vi "videoAQ.vi"() -> ()   [LabVIEW 2017]
doc: "This software allows video and synchronized audio acquisition. It allows video writing to be triggered manually, by a signal to a GPIO pin on the camera, or through audio volume levels."
uses:
  <vilib>/userdefined/High Color/IMAQdx.ctl
  <vilib>/vision/driver/IMAQdx.llb/IMAQdx Attribute Type.ctl
  <vilib>/vision/Image Controls.llb/IMAQ Image.ctl
  Mux paths.ctl
  Trigger message.ctl
  <vilib>/Utility/error.llb/DialogType.ctl
  <vilib>/vision/Avi.llb/IMAQ AVI2 Refnum.ctl
  <vilib>/sound2/lvsound2.llb/Sound File Refnum.ctl
  <vilib>/sound2/lvsound2.llb/Sound Data Format.ctl
  <vilib>/vision/driver/IMAQdx.llb/IMAQdx Attribute Visibility.ctl
  <vilib>/DAQmx/write.llb/DAQmx Write (Digital Bool 1Line 1Point).vi
  <vilib>/DAQmx/read.llb/DAQmx Read (Analog Wfm 1Chan NSamp).vi
  <vilib>/DAQmx/create/channels.llb/DAQmx Create Channel (DO-Digital Output).vi
  <vilib>/DAQmx/miscellaneous.llb/DAQmx Fill In Error Info.vi
  <vilib>/DAQmx/create/channels.llb/DAQmx Create Channel (AI-Voltage-Basic).vi
  <vilib>/DAQmx/configure/timing.llb/DAQmx Timing (Sample Clock).vi
  Latest DAQmx timestamp.vi
  <vilib>/sound2/lvsound2.llb/Sound File Write Open.vi
  <vilib>/vision/driver/NI_Vision_Acquisition_Software.lvlib
  <resource>/objmgr/imaqdx.rc
  <resource>/objmgr/daqmx.rc
panel:
  out "Events and errors":string
  in  "Audio chart":enum32{"Unfiltered audio", "Filtered audio"}(tab)
  out "Unfiltered audio":waveform(dbl)(graph)
  out "Filtered audio":waveform(dbl)(graph)
  in  "Toggle debug visibility":bool
  in  "Debugging stuff":enum32{"Debug monitoring", "Camera attributes"}(tab)
  out "New triggers sent":u32
  out "Write state":T1(ring)=enum."Stopped"
  out "Video capture state":T2(ring)=enum."Stopped"
  out "Audio capture state":T2(ring)=enum."Stopped"
  out "Mux loop state":enum16{"Waiting", "Muxing", "Exiting"}(ring)
  out "Trigger out state":T3(ring)
  out "UI event loop done":bool
  out "Trigger out loop done":bool
  out "Trigger detection loop done":bool
  out "Audio capture loop done":bool
  out "Camera capture loop done":bool
  out "Video write loop done":bool
  out "Mux loop done":bool
  out "STOP":bool=TRUE
  out "dt audio trigger loop":u32
  out "Mean under low threshold for required %":bool
  out "Mean above high threshold for required %":bool
  out "Current video trigger times":T4
  out "Audio file exists":bool
  out "Video file exists":bool
  out "Updated trigger list":T5(array[cluster])
  out "Trigger updates sent":u32
  out "detecting write trigger signal":errorcluster
  out "Error after closing AVI":errorcluster
  out "Error after closing WAV":errorcluster
  out "Error after sending paths to mux loop":errorcluster
  out "Muxing error":errorcluster
  out "Dequeuing mux path error":errorcluster
  out "concatenated string":string
  out "mux path cluster":T6
  out "Attribute Information Array":T8(array[cluster])
  in  "Main controls":enum32{"Page 1"}(tab) caption="Main\ncontrols"
  in  "stop button":bool
  in  "Trigger mode":enum16{"Manual", "GPIO", "Audio"}(ring)
  in  "Capture control":enum32{"Page 1"}(tab)
  in  "Capture":bool
  in  "Enable video capture":bool=TRUE caption="Video"
  in  "Enable audio capture":bool caption="Audio"
  in  "Write control":enum32{"Page 1"}(tab)
  in  "Enable audio write":bool caption="Audio"
  in  "Enable video write":bool=TRUE caption="Video"
  in  "Trigger write to file":bool
  in  "Status":enum32{"Page 2"}(tab)
  out "Acquire framerate (fps)":dbl
  out "Video buffer":dbl(slide) scale=0.0..100.0
  out "Video buffer\n size (s)":dbl format="%_3f"
  out "Missed Frames":bool
  out "Audio buffer\nsize (s)":dbl format="%_3f"
  out "Audio buffer":dbl(slide) scale=0.0..100.0
  out "Writing video":bool
  out "Writing audio":bool
  out "Acquire sample rate (Hz)":dbl
  out "Audio buffer size (frames)":i32=5000
  in  "Settings":T9(tab)
  in  "Estimated camera latency (s)":dbl=236.0
  in  "Select camera":T10="cam0"
  in  "Frames Per Second":dbl=30.0 min=2.0 max=120.0
  in  "Audio sample rate (Hz)":i64=44100
  in  "bits per sample":i32=16
  in  "Physical channel for audio input":tag="Dev2/ai0"
  in  "Samples per\nacquisition chunk":i32=1000
  in  "Delete audio file if \ncombining is successful?":bool=TRUE
  in  "Pre-trigger time* (s)":dbl=5.0 min=0.0
  in  "Record length* (s)":dbl=10.0 min=0.0
  out "Video buffer size (frames)":i32=5000
  in  "Write directory":path
  in  "Base Filename (no extension)":string
  in  "Video codec**":string(combo)="Microsoft Video 1"
  in  "Combine audio & \nvideo into one file*":bool=TRUE
  in  "GPIO line":string(combo)="Line 0"
  in  "Low Audio Threshold %":dbl=80.0 caption="...for this \n% of..." min=0.0 max=100.0 format="%0.1f"
  in  "High Audio Threshold %":dbl=10.0 caption="...for this \n% of..." min=0.0 max=100.0 format="%0.1f"
  in  "Low Audio Threshold":dbl=0.05 caption="If audio stays \nbelow this level..." format="%0.2f"
  in  "Time cutoff (s)":dbl=20.0 caption="No matter what, stop recording \nafter this amount of time (s)"
  in  "Low monitoring period (s)":dbl=10.0 caption="...this period of time (s),\nstop the recording"
  in  "Low cutoff freq (Hz)":dbl=1000.0 format="%0.3f"
  in  "High cutoff freq (Hz)":dbl=7000.0 format="%0.3f"
  in  "High monitoring period (s)":dbl=1.0 caption="...this period of time (s), \ntrigger a recording."
  in  "High Audio Threshold":dbl=0.2 caption="If audio stays \nabove this level..." format="%0.2f"
  out "Filtered audio amplitude":T11(graph)
  out "% above high threshold":dbl format="%#.1f%"
  out "% below low threshold":dbl format="%#.1f%"
  in  "Audio trigger enable":bool=TRUE
  in  "Physical channel for trigger out":tag="Dev2/ai0"
  in  "Enable trigger out":bool
  out "Trigger out":bool
  out "Current camera session reference":T10
  out "Video input":T12(plugin-control)
  # "Video Acquisition"
  # "This is the estimated time between the camera taking an image and transmitting it to the computer. This can correct for camera latency related desyncing of audio and video."
  # "To maintain video and audio in sync, samples per acquisition * video framerate should be smaller than audio sample rate."
  # "*Applies to manual \nand GPIO trigger modes"
  # "*Requires ffmpeg"
  # "**Recommended codec:\nMicrosoft Video 1"
  # ".avi"
  # ".wav"
  # "Settings for triggering write based on GPIO input pins on the camera \n(probably will only work for Pt Grey cameras like the Flea3)"
  # "Trigger pulse should be:\n - Positive polarity (0V normally, 5V during trigger pulse)\n - At least 1/f seconds long, where f = framerate.\n - Recording will start within 1/f of the trigger receive time."
  # "Settings for triggering write based on filtered audio volume"
  # "Bandpass filter cutoffs for audio before measuring volume for triggering"
  # "Send a digital trigger out to other devices for synchronization"
  # "Trigger signal with be digital ON between recording trigger time and recording stop time, \nand digital OFF otherwise. Note that trigger signal is not ON during pre-trigger recording time."
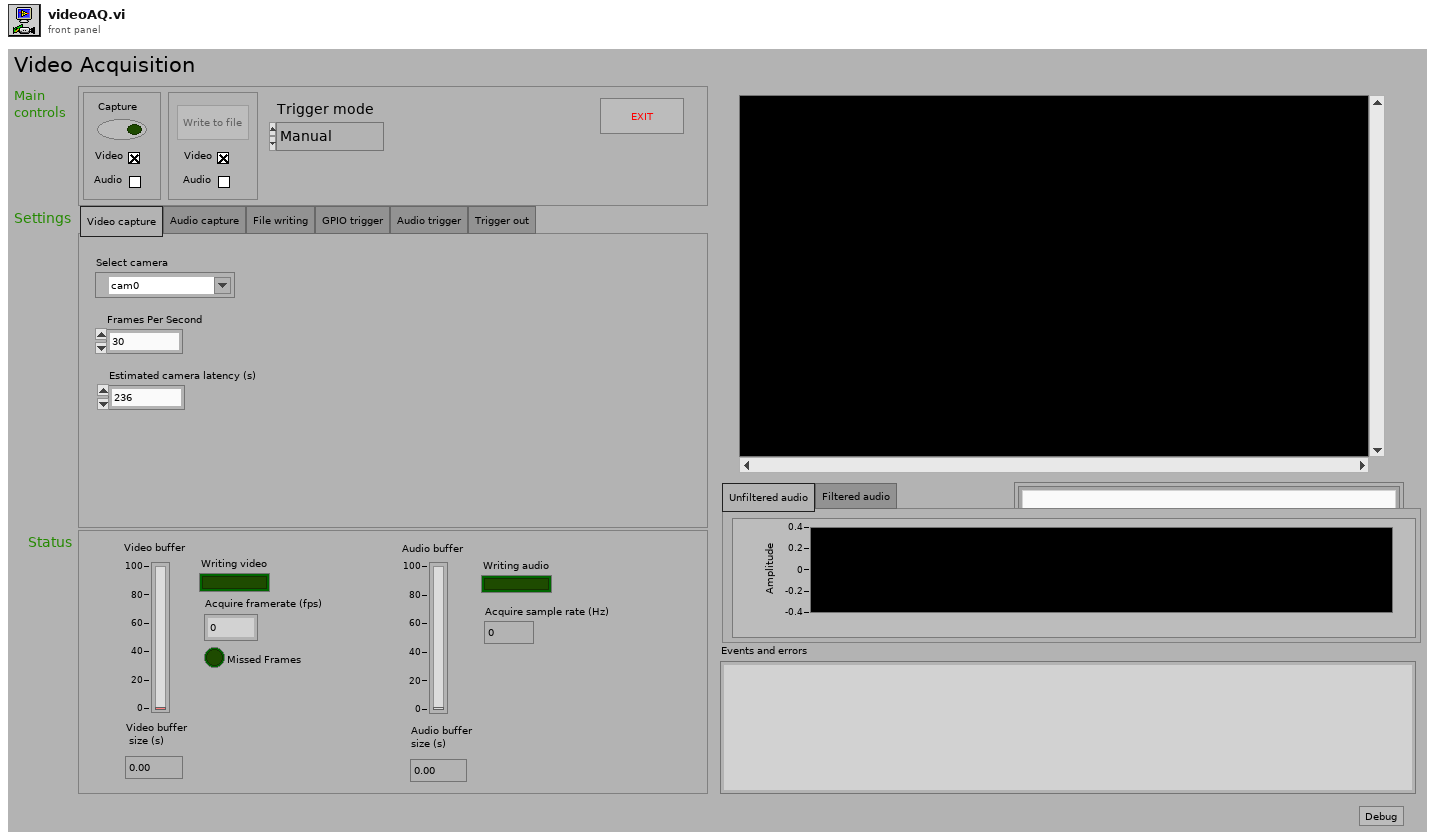
[diagram p1: front panel]
types:
  T1 = enum16{"Initializing", "Saving", "Closing file", "Stopped", "Paused", "Exiting"}
  T2 = enum16{"Initializing", "Capturing", "Stopping", "Stopped", "Exiting"}
  T3 = enum16{"Stopped", "Initializing", "Sending trigger", "Stopping", "Exiting"}
  T4 = cluster{"Start time":timestamp, "Trigger time":timestamp, "End time":timestamp}
  T5 = cluster{"Start time":timestamp, "Trigger time":timestamp, "End time":timestamp}[]
  T6 = cluster{"Available file path":path, "Available file path":path}
  T7 = typedef "NI_Vision_Acquisition_Software.lvlib/IMAQdx Attribute Type.ctl" = enum32{"U32", "I64", "DBL", "String", "Enum", "Bool", "Command"}
  T8 = cluster{"Attribute Type":T7, "Readable":bool, "Writable":bool, "Attribute Name":string}[]
  T9 = enum32{"Video capture", "Audio capture", "File writing", "GPIO trigger", "Audio trigger", "Trigger out"}
  T10 = typedef "IMAQdx.ctl" = refnum<k21>
  T11 = cluster{"Amplitude":dbl, "High Audio Threshold":dbl, "Low Audio Threshold":dbl}
  T12 = typedef "IMAQ Image.ctl" = refnum<image>
  T13 = typedef "Mux paths.ctl" = cluster{"Video path":path, "Audio path":path}
  T14 = typedef "Trigger message.ctl" = enum16{"New trigger", "Updated trigger"}
  T15 = cluster{"Trigger timestamps":cluster{"Start time":timestamp, "Trigger time":timestamp, "End time":timestamp}, "Message type":T14}
  T16 = enum16{"Always On", "Always Off", "Off While Running"}
  T17 = enum16{"At or before start", "In range", "At or after end"}
  T18 = enum16{"Stopped", "Initializing", "Sending trigger", "Stopping"}
  T19 = typedef "DialogType.ctl" = u16
  T20 = typedef "NI_Vision_Acquisition_Software.lvlib/IMAQdx Attribute Visibility.ctl" = enum32{"Simple", "Intermediate", "Advanced"}
  T21 = enum8{"Enabled", "Disabled", "Disabled and Grayed Out"}
  T22 = enum32{"Page Enabled", "Page Disabled", "Page Disabled & Grayed"}
  T23 = typedef "IMAQ AVI2 Refnum.ctl" = refnum<k20>
  T24 = typedef "Sound File Refnum.ctl" = refnum<file>
  T25 = typedef "Sound Data Format.ctl" = cluster{"sample rate (S/s)":dbl, "number of channels":i32, "bits per sample":i32}
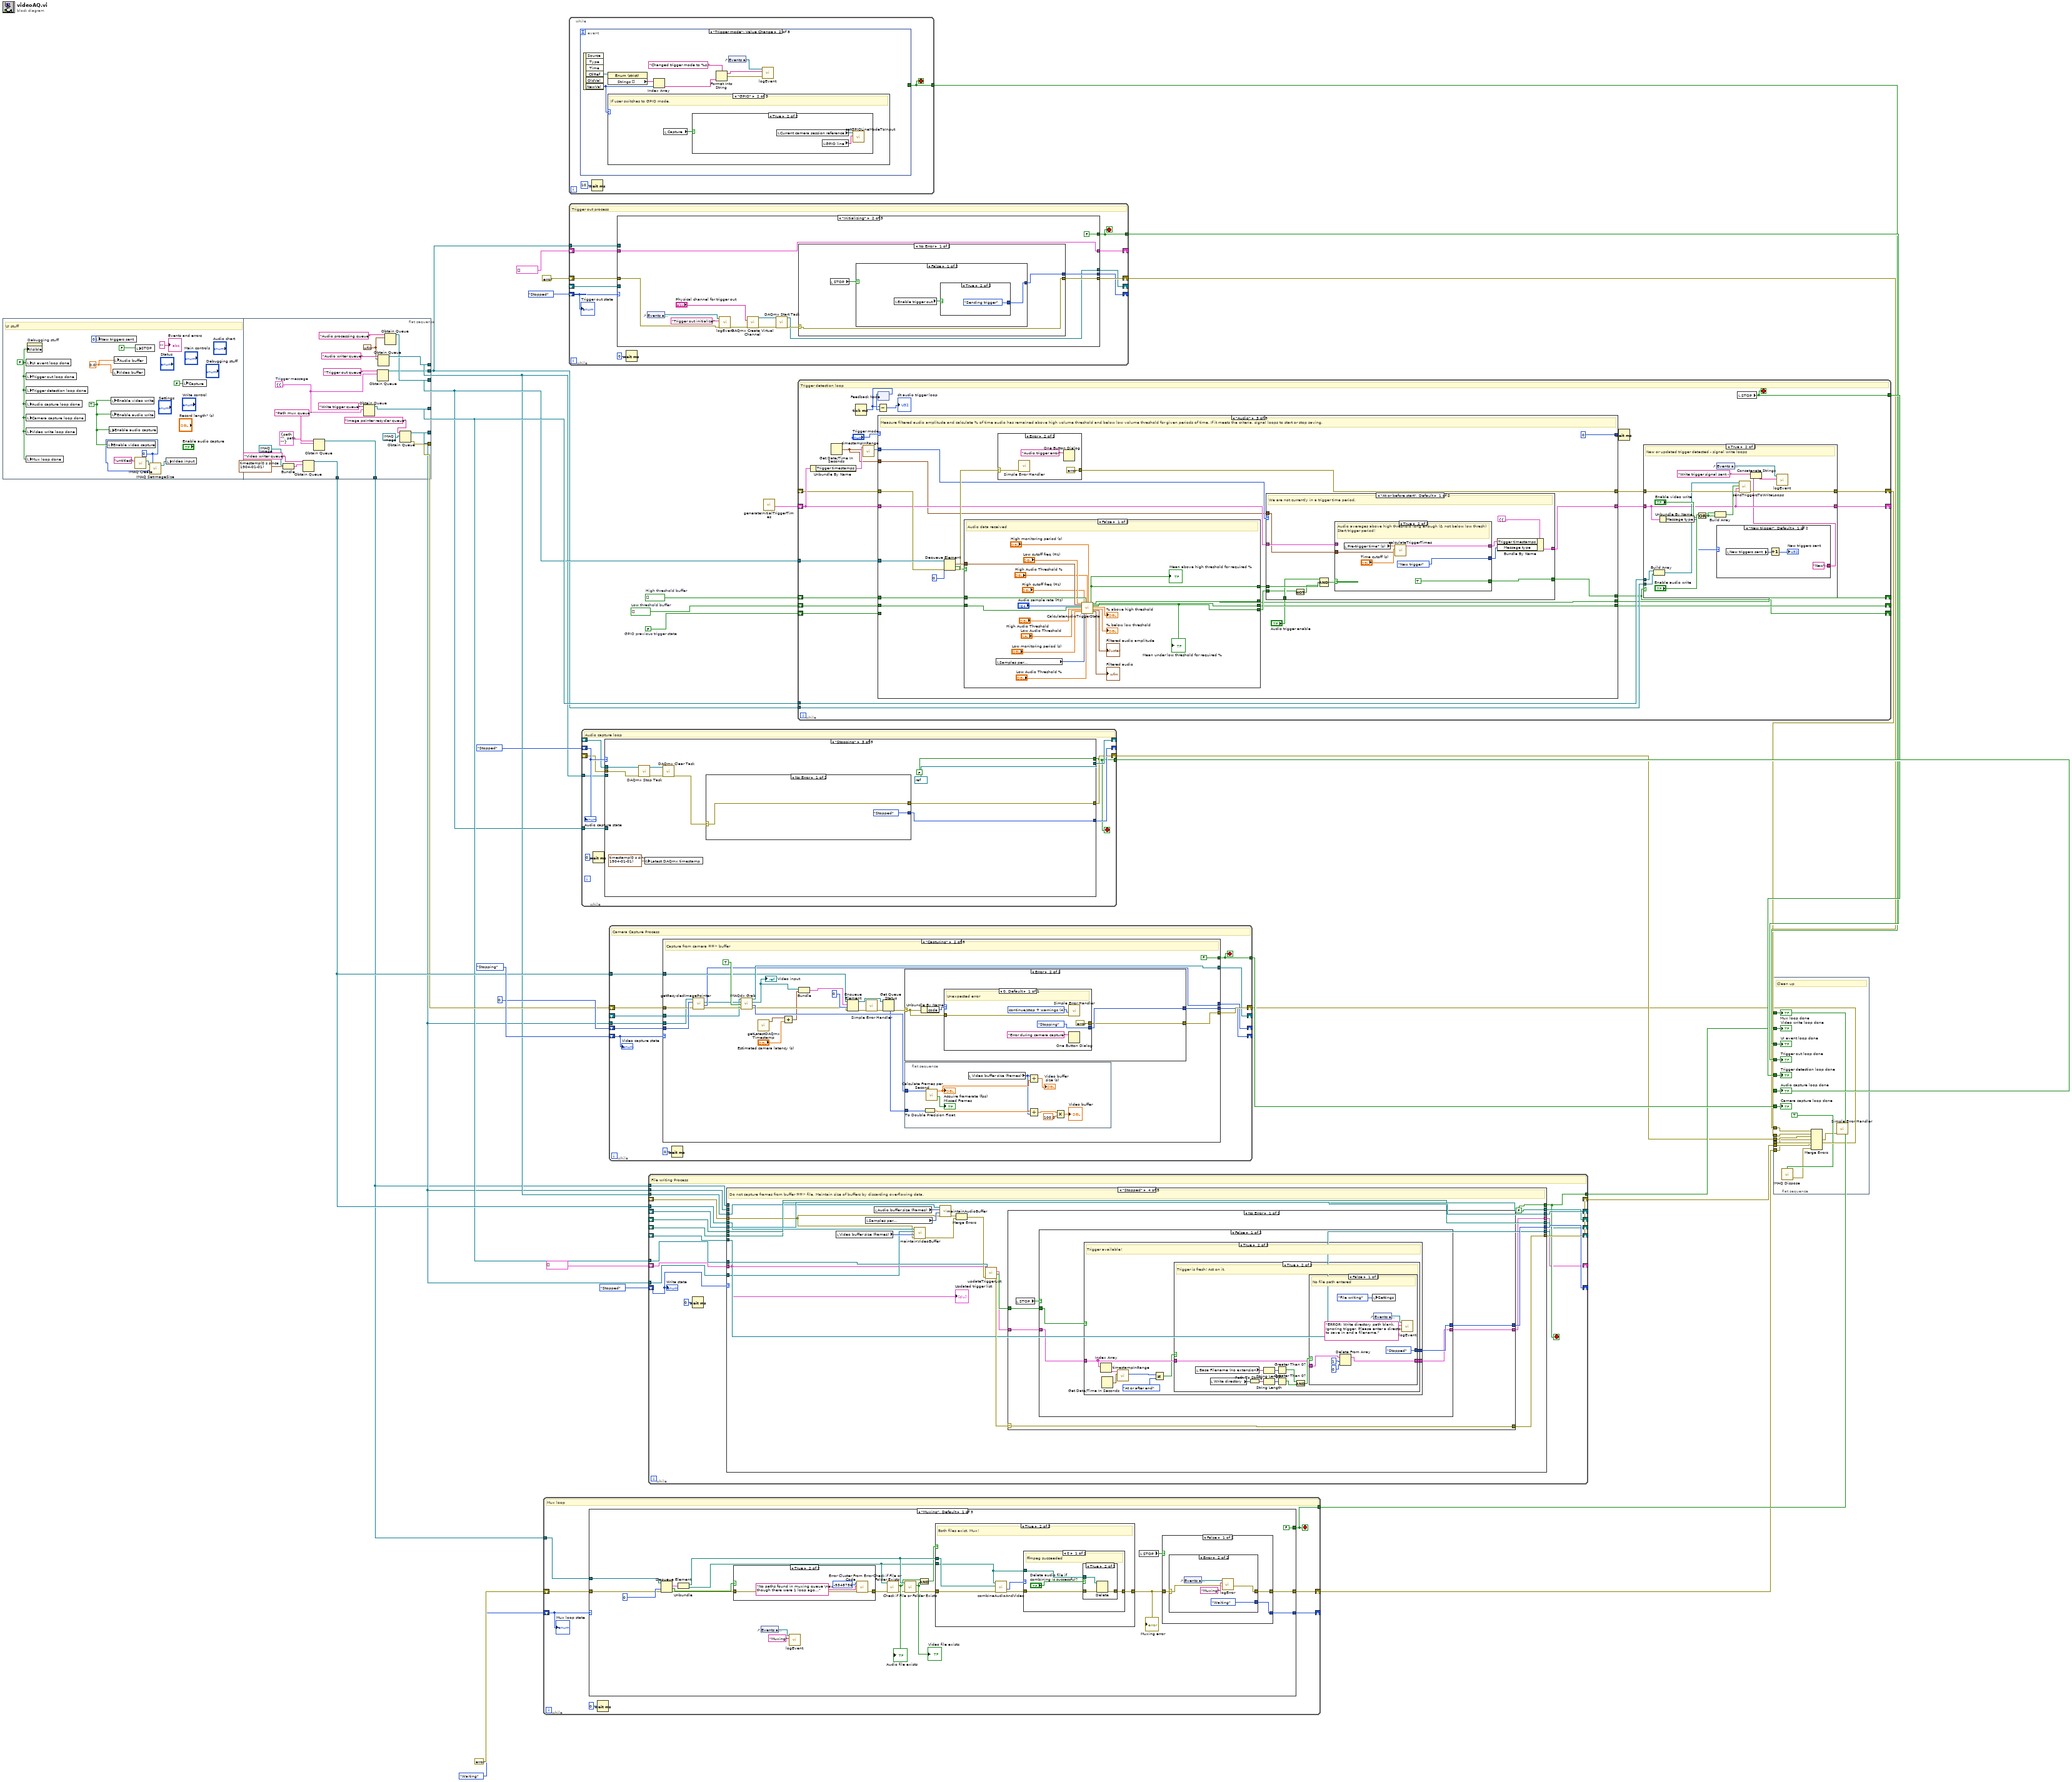
[diagram p0: block diagram]
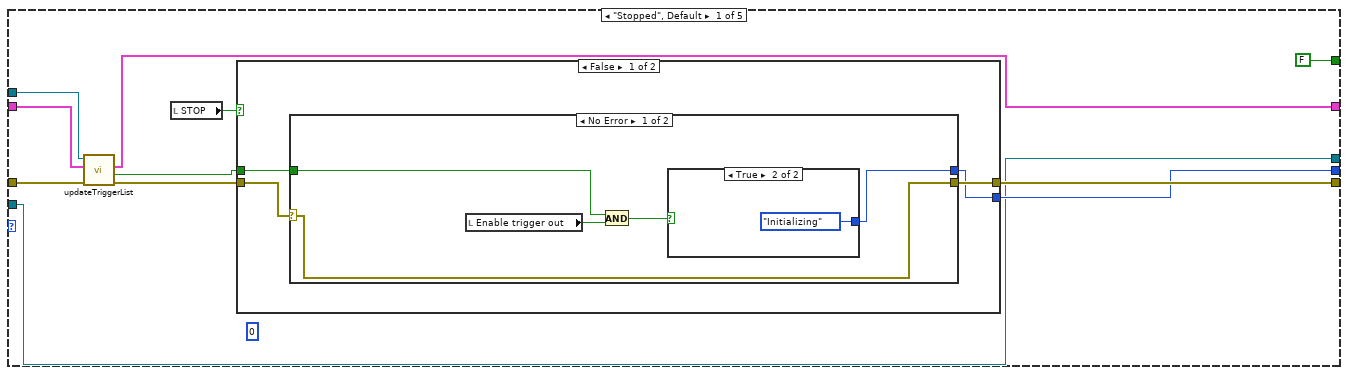
[diagram p2: hidden frame]
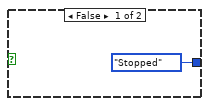
[diagram p3: hidden frame]
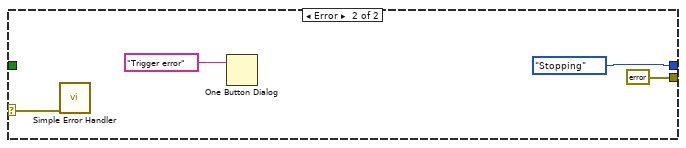
[diagram p4: hidden frame]
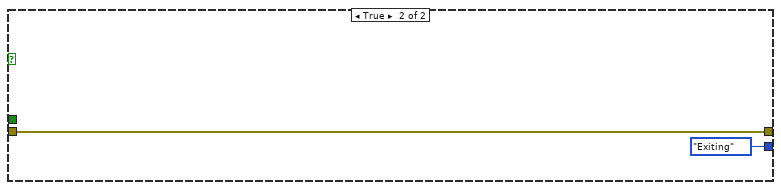
[diagram p5: hidden frame]
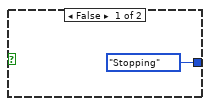
[diagram p6: hidden frame]
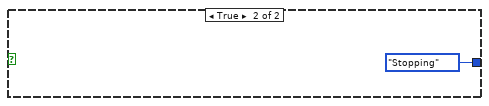
[diagram p7: hidden frame]
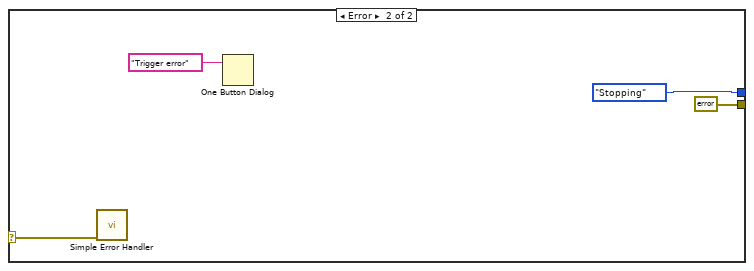
[diagram p8: hidden frame]
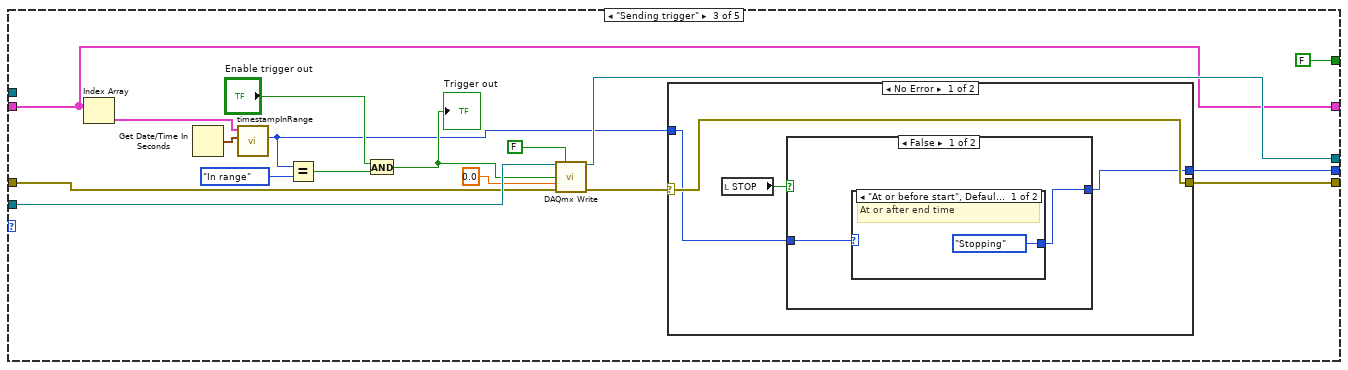
[diagram p9: hidden frame]
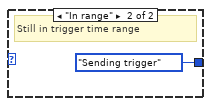
[diagram p10: hidden frame]
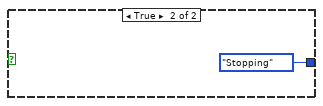
[diagram p11: hidden frame]
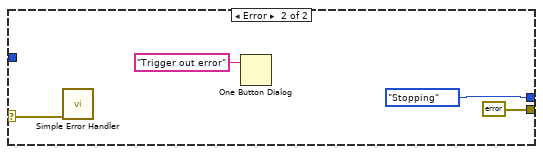
[diagram p12: hidden frame]
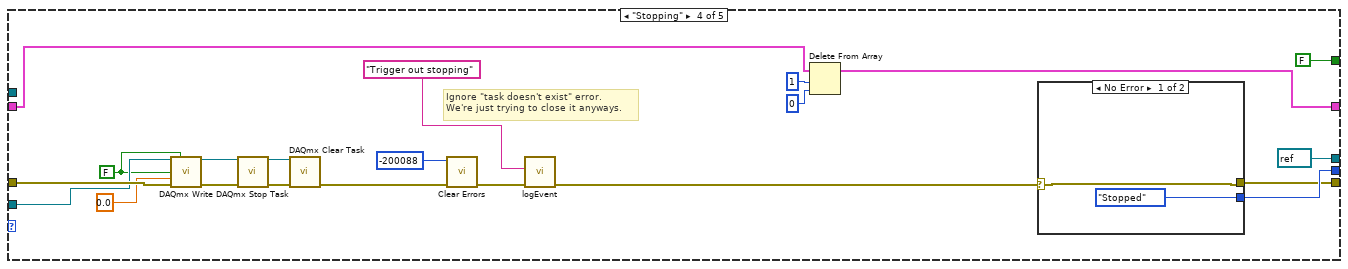
[diagram p13: hidden frame]
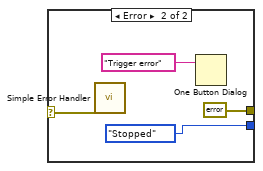
[diagram p14: hidden frame]
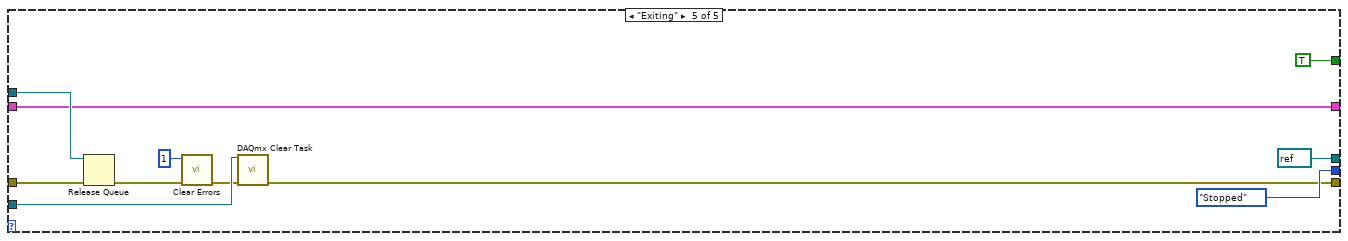
[diagram p15: hidden frame]
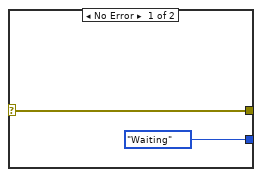
[diagram p17: hidden frame]
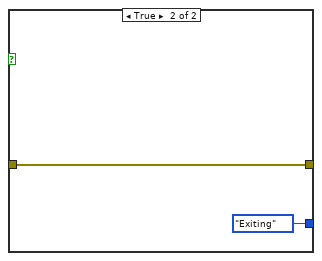
[diagram p18: hidden frame]
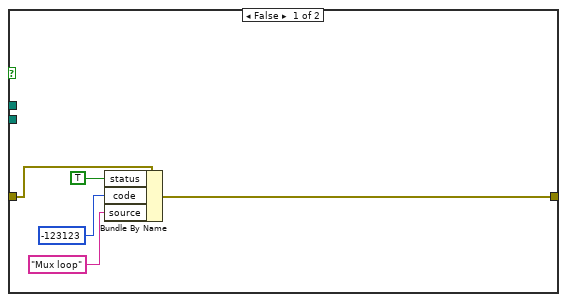
[diagram p19: hidden frame]
diagram:
  w23 = FALSE  # GPIO previous trigger state
  w24 = bool[] []  # Low threshold buffer
  w25 = bool[] []  # High threshold buffer
  n1 = flat-sequence {
    tunnel: [w66] -> w33
    tunnel: [w62] -> w31
    tunnel: [w61] -> w6
    tunnel: [w59] -> w7
    tunnel: [w57] -> w28
    tunnel: [w55] -> w29
    tunnel: [w53] -> w2
    tunnel: [w49] -> w26
    frame #0 {
      w37 = FALSE ("UI event loop done")
      w42 = 0 ("X Resolution")
      w44 = 0.0 ("Audio buffer")
      w45 = TRUE
      # "UI stuff"
      n2 = local write "UI event loop done"(w37) -> ()
      n3 = local write "Trigger out loop done"(w37) -> ()
      n4 = local write "Trigger detection loop done"(w37) -> ()
      n5 = local write "Audio capture loop done"(w37) -> ()
      n6 = local write "Camera capture loop done"(w37) -> ()
      n7 = local write "Video write loop done"(w37) -> ()
      n8 = local write "Mux loop done"(w37) -> ()
      n9 = property on="Debugging stuff" class="TabCtl (strict)"("Visible"=w37) -> ()  [unwired: 2 in, 2 out]
      n10 = local write "New triggers sent"(u32 0 ("Triggers sent")) -> ()
      n11 = local write "Enable video capture"(w45) -> ()
      n12 = local write "Enable audio capture"(w45) -> ()
      n13 = local write "Enable video write"(w45) -> ()
      n14 = local write "Enable audio write"(w45) -> ()
      n15 = local write "Video buffer"(w44) -> ()
      n16 = local write "Audio buffer"(w44) -> ()
      n17 = call "IMAQ Create"("Image Name"="untitled") -> ("New Image"=w41:T12)  [unwired: 3 in, 2 out]
      n18 = local write "STOP"(FALSE ("STOP SIGNAL")) -> ()
      n19 = call "IMAQ SetImageSize"("Y Resolution"=w42, "X Resolution"=w42, "Image"=w41) -> ("Image Out"=w40:T12)  [unwired: 2 in, 1 out]
      n20 = local write "Video input"(w40) -> ()
      n21 = local write "Capture"(FALSE ("Capture")) -> ()
      "Events and errors" <- "" ("Events and errors")
    }
    frame #1 {
      w47 = T15 {"Trigger timestamps"={"Start time"=timestamp(0 s since 1904-01-01), "Trigger time"=timestamp(0 s since 1904-01-01), "End time"=timestamp(0 s since 1904-01-01)}, "Message type"=enum."New trigger"}  # Trigger message
      w50 = waveform(dbl) {"t0"=timestamp(0 s since 1904-01-01), "dt"=1.0, "Y"=[]} ("element")
      n22 = Bundle("Image Out"=T12 refnum, timestamp(0 s since 1904-01-01)) -> (w65:cluster{"Image Out":T12, timestamp})  [unwired: 1 in]
      n23 = Obtain Queue(name (unnamed)="Video writer queue", element data type=w65) -> (queue out=w66:refnum<queue>)  [unwired: 3 in, 2 out]
      n24 = Obtain Queue(name (unnamed)="Path mux queue", element data type=T13 {"Video path"=path "", "Audio path"=path ""} ("cluster")) -> (queue out=w53:refnum<queue>)  [unwired: 3 in, 2 out]
      n25 = Obtain Queue(name (unnamed)="Write trigger queue", element data type=w47) -> (queue out=w55:refnum<queue>)  [unwired: 3 in, 2 out]
      n26 = Obtain Queue(name (unnamed)="Trigger out queue", element data type=w47) -> (queue out=w49:refnum<queue>)  [unwired: 3 in, 2 out]
      n27 = Obtain Queue(name (unnamed)="Audio writer queue", element data type=w50) -> (queue out=w59:refnum<queue>)  [unwired: 3 in, 2 out]
      n28 = Obtain Queue(name (unnamed)="Audio processing queue", element data type=w50) -> (queue out=w57:refnum<queue>)  [unwired: 3 in, 2 out]
      n29 = Obtain Queue(name (unnamed)="Image pointer recycler queue", element data type=T12 refnum ("Image Out")) -> (queue out=w61:refnum<queue>, error out=w62:errorcluster)  [unwired: 3 in, 1 out]
    }
  }
  n30 = while {
    shift-right: [w74] -> w8
    shift-left: errorcluster {"status"=FALSE, "code"=0, "source"=""} ("error IO") -> [w75]
    shift-right: [w71] -> _
    shift-left: enum16{"Waiting", "Muxing", "Exiting"}."Waiting" -> [w72]
    tunnel: [w70] -> w14
    tunnel: w2 -> [w69]
    stop <- w70 stop-if-true
    # "Mux loop"
    n31 = case shown="\"Muxing\", Default" w72 {
      tunnel: w75 -> [w78 w142 w163]
      tunnel: [w95 w146 errorcluster {"status"=FALSE, "code"=0, "source"=""} ("error IO")] -> w74
      tunnel: w69 -> [w88 w145 w165]
      tunnel: [w87 w140 enum16{"Waiting", "Muxing", "Exiting"}."Exiting"] -> w71
      tunnel: [FALSE FALSE TRUE] -> w70
      frame "Muxing", Default {
        n32 = Dequeue Element(queue=w88, timeout in ms (-1)=0, error in (no error)=w78) -> (element=w93:T13, timed out?=w80:bool, error out=w94:errorcluster)  [unwired: 1 out]
        n33 = Unbundle(w93) -> ("Video path"=w92:path, "Audio path"=w79:path)
        n34 = case shown="True" w80 {
          tunnel: w94 -> [w97 w101]
          tunnel: [w97 w100] -> w82
          frame False {
          }
          frame True {
            n35 = call <vilib>:"Error Cluster From Error Code.vi"("error in (no error)"=w101, "error message (\"\")"="No paths found in muxing queue \neven though there were 1 loop ago..." ("error message (\"\")"), "error code (0)"=-9348756) -> ("error out"=w100:errorcluster)  [unwired: 6 in]
          }
        }
        n36 = control-ref of="Events and errors"() -> (w76:refnum<vi>)
        n37 = call "logEvent.vi"("New log entry"="Muxing", "Text reference"=w76) -> ()  [unwired: 9 in, 1 out]
        n38 = call <vilib>:"Check if File or Folder Exists.vi"("error in (no error)"=w82, "path"=w79) -> ("error out"=w89:errorcluster, "file or folder exists?"=w90:bool)  [unwired: 7 in, 1 out]
        "Audio file exists" <- w90
        n39 = call <vilib>:"Check if File or Folder Exists.vi"("error in (no error)"=w89, "path"=w92) -> ("error out"=w81:errorcluster, "file or folder exists?"=w91:bool)  [unwired: 7 in, 1 out]
        "Video file exists" <- w91
        n40 = And(x=w90, y=w91) -> (x .and. y?=w85:bool)
        n41 = case shown="True" w85 {
          tunnel: w81 -> [w117 w124]
          tunnel: [w118 w120] -> w96
          tunnel: w92 -> [_ w123]
          tunnel: w79 -> [_ w119]
          frame False {
            n42 = Bundle By Name(cluster=w117, "status"=TRUE, "code"=-123123, "source"="Mux loop") -> (w118:errorcluster)
          }
          frame True {
            # "Both files exist. Mux!"
            n43 = call "combineAudioAndVideo.vi"("error in (no error)"=w124, "Video path"=w123, "Audio path"=w119) -> ("error out"=w121:errorcluster, "return code"=w122:i32)  [unwired: 7 in]
            n44 = case shown="0" w122 {
              selector: w122 -> [_ w136]
              tunnel: w121 -> [w126 w134]
              tunnel: [w125 w133] -> w120
              tunnel: w119 -> [w127 _]
              frame 0 {
                # "ffmpeg succeeded"
                n45 = case shown="True" "Delete audio file if \ncombining is successful?" {
                  tunnel: w127 -> [_ w132]
                  tunnel: w126 -> [w129 w131]
                  tunnel: [w129 w130] -> w125
                  frame False {
                  }
                  frame True {
                    n46 = Delete(path (use dialog)=w132, error in=w131) -> (error out=w130:errorcluster)  [unwired: 3 in, 2 out]
                  }
                }
              }
              frame -1, Default {
                # "ffmpeg did not succeed"
                n47 = call <vilib>:"Error Cluster From Error Code.vi"("error in (no error)"=w134, "error message (\"\")"="ffmpeg error" ("error message (\"\")"), "error code (0)"=w136) -> ("error out"=w133:errorcluster)  [unwired: 6 in]
              }
            }
          }
        }
        "Muxing error" <- w96
        n48 = local read "STOP"() -> (w84:bool)
        n49 = case shown="False" w84 {
          tunnel: w96 -> [w104 w112]
          tunnel: [w103 w112] -> w95
          tunnel: [w102 enum16{"Waiting", "Muxing", "Exiting"}."Exiting"] -> w87
          frame False {
            n50 = case shown="Error" w104 {
              selector: w104 -> [w106 w108]
              tunnel: [w106 w107] -> w103
              tunnel: [enum16{"Waiting", "Muxing", "Exiting"}."Waiting" enum16{"Waiting", "Muxing", "Exiting"}."Waiting"] -> w102
              frame No Error {
              }
              frame Error {
                n51 = control-ref of="Events and errors"() -> (w109:refnum<vi>)
                n52 = call "logError.vi"("Error to log"=w108, "Location"="Muxing", "Text reference"=w109) -> ("error out"=w107:errorcluster)  [unwired: 8 in]
              }
            }
          }
          frame True {
          }
        }
      }
      frame "Waiting" {
        # "Ignore error due to invalid queue"
        n53 = Get Queue Status(queue=w145, error in (no error)=w142) -> (error out=w138:errorcluster, # elements in queue=w144:i32)  [unwired: 1 in, 6 out]
        n54 = Greater Than 0?(x=w144) -> (x > 0?=w143:bool)
        n55 = call <vilib>:"Clear Errors.vi"("error in (no error)"=w138, "specific error code to clear (0: all)"=1) -> ("error out"=w139:errorcluster)  [unwired: 4 in, 1 out]
        "Dequeuing mux path error" <- w139
        n56 = case shown="Error" w139 {
          selector: w139 -> [w150 w157]
          tunnel: [w150 w156] -> w146
          tunnel: [w148 enum16{"Waiting", "Muxing", "Exiting"}."Waiting"] -> w140
          tunnel: w143 -> [w149 _]
          frame No Error {
            n57 = local read "STOP"() -> (w147:bool)
            n58 = case shown="False" w147 {
              tunnel: w149 -> [w152 _]
              tunnel: [w151 enum16{"Waiting", "Muxing", "Exiting"}."Exiting"] -> w148
              frame False {
                n59 = case shown="False" w152 {
                  tunnel: [enum16{"Waiting", "Muxing", "Exiting"}."Waiting" enum16{"Waiting", "Muxing", "Exiting"}."Muxing"] -> w151
                  frame False {
                    # "Haven't received audio and \nvideo paths yet. Continue waiting"
                  }
                  frame True {
                    # "Audio and video file paths received.\nBegin muxing!"
                  }
                }
              }
              frame True {
              }
            }
          }
          frame Error {
            n60 = control-ref of="Events and errors"() -> (w158:refnum<vi>)
            n61 = call "logError.vi"("Error to log"=w157, "Location"="Mux waiting", "Text reference"=w158) -> ("error out"=w156:errorcluster)  [unwired: 8 in]
          }
        }
      }
      frame "Exiting" {
        (unwired) refnum<queue> refnum ("queue out")
        n62 = Release Queue(queue=w165, force destroy? (F)=FALSE, error in (no error)=w163) -> ()  [unwired: 3 out]
      }
    }
    n63 = Wait (ms)(milliseconds to wait=u32 0) -> ()  [unwired: 1 out]
    "Mux loop state" <- w72
  }
  n64 = while {
    tunnel: [w167] -> w16
    stop <- w167 stop-if-true
    n65 = event shown="[1] \"Trigger mode\": Value Change" {
      selector: _ -> [_ _ _ _ _ _ _ _]
      dyn-events: _ -> [_ _ _ _ _ _ _ _]
      timeout: _ -> [_ _ _ _ _ _ _ _]
      tunnel: [_ _ _ w187 _ _ _ _] -> w167
      event "Enable video capture": Value Change {
        n66 = event-data() -> ("NewVal"=w169:bool)  [unwired: 1 in, 5 out]
        n67 = case shown="False" w169 {
          frame False {
            n68 = local write "Enable video write"(FALSE ("Enable video write")) -> ()
            n69 = local write "Enable audio capture"(TRUE ("Enable audio capture")) -> ()
          }
          frame True {
          }
        }
      }
      event "Trigger mode": Value Change {
        n70 = event-data() -> ("CtlRef"=w179:refnum<vi>, "NewVal"=w177:enum16{"Manual", "GPIO", "Audio"})  [unwired: 1 in, 4 out]
        n71 = property class="Enum (strict)"(reference=w179) -> ("Strings []"=w178:string[])  [unwired: 1 in, 2 out]
        n72 = case shown="\"GPIO\"" w177 {
          frame "Manual", Default {
          }
          frame "GPIO" {
            # "If user switches to GPIO mode,"
            n73 = local read "Capture"() -> (w180:bool)
            n74 = case shown="True" w180 {
              frame False {
              }
              frame True {
                n75 = local read "Current camera session reference"() -> (w182:T10)
                n76 = local read "GPIO line"() -> (w181:string)
                n77 = call "setGPIOLineModeToInput.vi"("GPIO line"=w181, "IMAQdx Session in"=w182) -> ()  [unwired: 8 in, 2 out]
              }
            }
          }
          frame "Audio" {
            n78 = local write "Enable audio capture"(TRUE ("Enable audio capture")) -> ()
          }
        }
        n79 = Index Array(array=w178, index=w177) -> (element=w173:string)
        n80 = Format Into String(format string="Changed trigger mode to %s.", w173) -> (resulting string=w175:string, error out=w174:errorcluster)  [unwired: 2 in]
        n81 = control-ref of="Events and errors"() -> (w172:refnum<vi>)
        n82 = call "logEvent.vi"("error in (no error)"=w174, "New log entry"=w175, "Text reference"=w172) -> ()  [unwired: 8 in, 1 out]
      }
      event "High Audio Threshold": Value Change {
        n83 = event-data() -> ("NewVal"=w186:dbl)  [unwired: 1 in, 5 out]
        n84 = Multiply(x=1.5, y=w186) -> (x*y=w184:dbl)
        n85 = property on="Filtered audio amplitude" class="WFChart (strict)"("YScale.Maximum"=w184) -> ()  [unwired: 2 in, 2 out]
      }
      event "stop button": Value Change {
        n86 = event-data() -> ()  [unwired: 1 in, 6 out]
        n87 = case shown="True" "stop button" {
          tunnel: [FALSE ("STOP SIGNAL") w190] -> w187
          frame False {
          }
          frame True {
            w190 = TRUE ("STOP SIGNAL")
            # "Set stop signal to true"
            "STOP" <- w190
          }
        }
      }
      event "Toggle debug visibility": Value Change {
        n88 = event-data() -> ()  [unwired: 1 in, 6 out]
        n89 = property on="Debugging stuff" class="TabCtl (strict)"() -> ("Visible"=w197:bool)  [unwired: 2 in, 2 out]
        n90 = Not(x=w197) -> (.not. x?=w192:bool)
        n91 = case shown="False" w192 {
          tunnel: [T16."Always Off" ("Horizontal Scrollbar Visibility") T16."Always On" ("Horizontal Scrollbar Visibility")] -> w191
          frame False {
          }
          frame True {
          }
        }
        n92 = property on="Debugging stuff" class="TabCtl (strict)"("Visible"=w192) -> ()  [unwired: 2 in, 2 out]
        n93 = property class="VI"() -> ("Panel"=w194:refnum<vi>)  [unwired: 2 in, 2 out]
        n94 = property class="Pnl"(reference=w194) -> ("Panes[]"=w195:refnum<vi>[])  [unwired: 1 in, 2 out]
        n95 = Index Array(array=w195) -> (element=w196:refnum<vi>)  [unwired: 1 in]
        n96 = property class="Pane"(reference=w196, "HorizScrollbarVisibility"=w191) -> ()  [unwired: 1 in, 2 out]
        n97 = property class="Pane"(reference=w196, "VertScrollbarVisibility"=w191) -> (reference out=w193:refnum<vi>)  [unwired: 1 in, 1 out]
        n98 = Close Reference(reference=w193) -> ()  [unwired: 1 in, 1 out]
      }
      event "Enable audio capture": Value Change {
        n99 = event-data() -> ("NewVal"=w200:bool)  [unwired: 1 in, 5 out]
        n100 = case shown="False" w200 {
          frame False {
            n101 = local write "Enable audio write"(FALSE ("Enable video write")) -> ()
            n102 = local write "Enable video capture"(TRUE ("Enable video capture")) -> ()
          }
          frame True {
          }
        }
      }
      event "Enable video write": Value Change {
        n103 = event-data() -> ("NewVal"=w203:bool)  [unwired: 1 in, 5 out]
        n104 = case shown="True" w203 {
          frame False {
            n105 = local write "Enable audio write"(TRUE ("Enable audio write")) -> ()
          }
          frame True {
            n106 = local write "Enable video capture"(TRUE ("Enable video capture")) -> ()
          }
        }
      }
      event "Enable audio write": Value Change {
        n107 = event-data() -> ("NewVal"=w206:bool)  [unwired: 1 in, 5 out]
        n108 = case shown="True" w206 {
          frame False {
            # "If audio write is set to false, set video write to true"
            n109 = local write "Enable video write"(TRUE ("Enable video write")) -> ()
          }
          frame True {
            # "If audio write is set to true, set audio capture to true too"
            n110 = local write "Enable audio capture"(TRUE ("Enable audio capture")) -> ()
          }
        }
      }
    }
    n111 = Wait (ms)(milliseconds to wait=u32 10) -> ()  [unwired: 1 out]
  }
  n112 = while {
    shift-right: [w218] -> w13
    shift-left: errorcluster {"status"=FALSE, "code"=0, "source"=""} ("error IO") -> [w219]
    shift-right: [w217] -> _
    shift-left: _ -> [w216]
    tunnel: w26 -> [w215]
    shift-right: [w209] -> _
    shift-left: T5 [] -> [w210]
    shift-right: [w212] -> _
    shift-left: T3."Stopped" -> [w213]
    tunnel: [w211] -> w17
    stop <- w211 stop-if-true
    # "Trigger out process"
    n113 = case shown="\"Initializing\"" w213 {
      tunnel: w219 -> [w223 w251 w287 w315 w337]
      tunnel: [w230 w259 w285 w322 w334] -> w218
      tunnel: [w229 w260 w284 w323 T3."Stopped"] -> w212
      tunnel: [w228 w254 w288 refnum<k21> refnum ("task out") refnum<k21> refnum ("task out")] -> w217
      tunnel: w216 -> [w228 _ w289 w313 w336]
      tunnel: w215 -> [w224 _ _ _ w338]
      tunnel: [FALSE FALSE FALSE FALSE TRUE] -> w211
      tunnel: w210 -> [w225 w252 w280 w307 w330]
      tunnel: [w220 w252 w280 w306 w330] -> w209
      frame "Stopped", Default {
        (unwired) 0 ("timeout in ms (-1)")
        n114 = call "updateTriggerList.vi"("error in (no error)"=w223, "Trigger list"=w225, "Trigger queue in"=w224) -> ("error out"=w221:errorcluster, "Trigger available?"=w222:bool, "Updated trigger list"=w220:T5)  [unwired: 5 in, 1 out]
        n115 = local read "STOP"() -> (w226:bool)
        n116 = case shown="False" w226 {
          tunnel: [w234 w246] -> w230
          tunnel: [w233 T3."Exiting"] -> w229
          tunnel: w222 -> [w232 _]
          tunnel: w221 -> [w231 w246]
          frame False {
            n117 = case shown="No Error" w231 {
              selector: w231 -> [w239 w245]
              tunnel: [w239 errorcluster {"status"=FALSE, "code"=0, "source"=""} ("error IO")] -> w234
              tunnel: [w238 T3."Stopping"] -> w233
              tunnel: w232 -> [w235 _]
              frame No Error {
                n118 = local read "Enable trigger out"() -> (w237:bool)
                n119 = And(x=w235, y=w237) -> (x .and. y?=w236:bool)
                n120 = case shown="True" w236 {
                  tunnel: [T3."Stopped" T3."Initializing"] -> w238
                  frame False {
                  }
                  frame True {
                  }
                }
              }
              frame Error {
                n121 = call <vilib>:"Simple Error Handler.vi"("error in (no error)"=w245) -> ()  [unwired: 4 in, 5 out]
                n122 = One Button Dialog(message="Trigger error") -> ()  [unwired: 1 in, 1 out]
              }
            }
          }
          frame True {
          }
        }
      }
      frame "Initializing" {
        n123 = control-ref of="Events and errors"() -> (w248:refnum<vi>)
        n124 = call "logEvent.vi"("error in (no error)"=w251, "New log entry"="Trigger out initialize", "Text reference"=w248) -> ("error out"=w250:errorcluster)  [unwired: 8 in]
        n125 = call-poly <vilib>:"DAQmx Create Virtual Channel.vi"("lines"="Physical channel for trigger out", "error in"=w250) -> ("task out"=w256:refnum<k21>, "error out"=w257:errorcluster)  [unwired: 12 in]
        n126 = call <vilib>:"DAQmx Start Task.vi"("task/channels in"=w256, "error in"=w257) -> ("task out"=w254:refnum<k21>, "error out"=w255:errorcluster)  [unwired: 12 in]
        n127 = case shown="No Error" w255 {
          selector: w255 -> [w263 w272]
          tunnel: [w263 errorcluster {"status"=FALSE, "code"=0, "source"=""} ("error IO")] -> w259
          tunnel: [w262 T3."Stopping"] -> w260
          frame No Error {
            n128 = local read "STOP"() -> (w261:bool)
            n129 = case shown="False" w261 {
              tunnel: [w265 T3."Stopping"] -> w262
              frame False {
                n130 = local read "Enable trigger out"() -> (w264:bool)
                n131 = case shown="True" w264 {
                  tunnel: [T3."Stopping" T3."Sending trigger"] -> w265
                  frame False {
                  }
                  frame True {
                  }
                }
              }
              frame True {
              }
            }
          }
          frame Error {
            n132 = call <vilib>:"Simple Error Handler.vi"("error in (no error)"=w272) -> ()  [unwired: 4 in, 5 out]
            n133 = One Button Dialog(message="Trigger error") -> ()  [unwired: 1 in, 1 out]
          }
        }
      }
      frame "Sending trigger" {
        n134 = Index Array(array=w280) -> (element=w279:T4)  [unwired: 1 in]
        n135 = Get Date/Time In Seconds() -> (seconds since 1Jan1904=w277:timestamp)
        n136 = call "timestampInRange.vi"("Time Stamp"=w277, "Start and end times"=w279) -> ("timeState"=w273:T17)  [unwired: 9 in]
        n137 = Equal?(x=w273, y=T17."In range") -> (x = y?=w274:bool)
        n138 = And(x="Enable trigger out", y=w274) -> (x .and. y?=w275:bool)
        "Trigger out" <- w275
        n139 = call-poly <vilib>:"DAQmx Write.vi"("task/channels in"=w289, "auto start"=FALSE, "data"=w275, "timeout"=0.0, "error in"=w287) -> ("task out"=w288:refnum<k21>, "error out"=w286:errorcluster)  [unwired: 8 in, 1 out]
        n140 = case shown="No Error" w286 {
          selector: w286 -> [w293 w302]
          tunnel: [w293 errorcluster {"status"=FALSE, "code"=0, "source"=""} ("error IO")] -> w285
          tunnel: [w292 T18."Stopping"] -> w284
          tunnel: w273 -> [w290 _]
          frame No Error {
            n141 = local read "STOP"() -> (w291:bool)
            n142 = case shown="False" w291 {
              tunnel: [w295 T3."Stopping"] -> w292
              tunnel: w290 -> [w294 _]
              frame False {
                n143 = case shown="\"At or before start\", Default" w294 {
                  tunnel: [T3."Stopping" T3."Sending trigger"] -> w295
                  frame "At or before start", Default {
                    # "At or after end time"
                  }
                  frame "In range" {
                    # "Still in trigger time range"
                  }
                }
              }
              frame True {
              }
            }
          }
          frame Error {
            n144 = call <vilib>:"Simple Error Handler.vi"("error in (no error)"=w302) -> ()  [unwired: 4 in, 5 out]
            n145 = One Button Dialog(message="Trigger out error") -> ()  [unwired: 1 in, 1 out]
          }
        }
      }
      frame "Stopping" {
        w311 = FALSE ("auto start")
        # "Ignore \"task doesn't exist\" error.\nWe're just trying to close it anyways."
        n146 = call-poly <vilib>:"DAQmx Write.vi"("task/channels in"=w313, "auto start"=w311, "data"=w311, "timeout"=0.0, "error in"=w315) -> ("task out"=w312:refnum<k21>, "error out"=w314:errorcluster)  [unwired: 8 in, 1 out]
        n147 = call <vilib>:"DAQmx Stop Task.vi"("task/channels in"=w312, "error in"=w314) -> ("task out"=w321:refnum<k21>, "error out"=w320:errorcluster)  [unwired: 12 in]
        n148 = call <vilib>:"DAQmx Clear Task.vi"("task in"=w321, "error in"=w320) -> ("error out"=w319:errorcluster)  [unwired: 13 in]
        n149 = call <vilib>:"Clear Errors.vi"("error in (no error)"=w319, "specific error code to clear (0: all)"=-200088) -> ("error out"=w304:errorcluster)  [unwired: 4 in, 1 out]
        n150 = call "logEvent.vi"("error in (no error)"=w304, "New log entry"="Trigger out stopping") -> ("error out"=w303:errorcluster)  [unwired: 9 in]
        n151 = Delete From Array(array=w307, length=1, index=0) -> (array with subset deleted=w306:T5)  [unwired: 1 out]
        n152 = case shown="No Error" w303 {
          selector: w303 -> [w325 w327]
          tunnel: [w325 errorcluster {"status"=FALSE, "code"=0, "source"=""} ("error IO")] -> w322
          tunnel: [T3."Stopped" T3."Stopped"] -> w323
          frame No Error {
          }
          frame Error {
            n153 = call <vilib>:"Simple Error Handler.vi"("error in (no error)"=w327) -> ()  [unwired: 4 in, 5 out]
            n154 = One Button Dialog(message="Trigger error") -> ()  [unwired: 1 in, 1 out]
          }
        }
      }
      frame "Exiting" {
        n155 = Release Queue(queue=w338, error in (no error)=w337) -> (error out=w335:errorcluster)  [unwired: 1 in, 2 out]
        n156 = call <vilib>:"Clear Errors.vi"("error in (no error)"=w335, "specific error code to clear (0: all)"=1) -> ("error out"=w332:errorcluster)  [unwired: 4 in, 1 out]
        n157 = call <vilib>:"DAQmx Clear Task.vi"("task in"=w336, "error in"=w332) -> ("error out"=w334:errorcluster)  [unwired: 13 in]
      }
    }
    n158 = Wait (ms)(milliseconds to wait=u32 0) -> ()  [unwired: 1 out]
    "Trigger out state" <- w213
  }
  n159 = while {
    tunnel: w7 -> [w346]
    shift-right: [w344] -> _
    shift-left: T2."Stopped" -> [w350]
    shift-right: [w345] -> w11
    shift-left: _ -> [w349]
    shift-right: [w348] -> _
    shift-left: _ -> [w347]
    tunnel: w28 -> [w343]
    tunnel: [w341] -> w19
    stop <- w341 stop-if-true
    # "Audio capture loop"
    n160 = Wait (ms)(milliseconds to wait=u32 0) -> ()  [unwired: 1 out]
    n161 = case shown="\"Stopping\"" w350 {
      tunnel: [FALSE FALSE FALSE FALSE TRUE] -> w341
      tunnel: w349 -> [w361 w404 w442 w458 w469]
      tunnel: [w360 w405 refnum<k21> refnum ("task out") refnum<k21> refnum ("task out") refnum<k21> refnum ("task out")] -> w348
      tunnel: w347 -> [_ w406 w443 _ _]
      tunnel: w346 -> [_ w403 _ _ w471]
      tunnel: [w351 w396 w440 w458 w468] -> w345
      tunnel: [w352 w397 w439 w457 T2."Exiting"] -> w344
      tunnel: w343 -> [_ w394 _ _ _]
      frame "Initializing", Default {
        w372 = 10083 items=["default"=-1, "RSE"=10083, "NRSE"=10078, "Differential"=10106, "Pseudodifferential"=12529] ("Terminal Configuration")
        w376 = 10123 items=["Finite Samples"=10178, "Continuous Samples"=10123, "Hardware Timed Single Point"=12522]  # Sample Mode
        n162 = local read "Audio sample rate (Hz)"() -> (w368:i64)
        n163 = call-poly <vilib>:"DAQmx Create Virtual Channel.vi"("maximum value"=10.0 ("Max Voltage"), "minimum value"=-10.0 ("Min Voltage"), "input terminal configuration"=w372, "physical channels"="Physical channel for audio input", "error in"=w361) -> ("task out"=w374:refnum<k21>, "error out"=w375:errorcluster)  [unwired: 9 in]
        n164 = call-poly <vilib>:"DAQmx Timing.vi"("task/channels in"=w374, "sample mode"=w376, "samples per channel"="Samples per\nacquisition chunk", "rate"=w368, "source"=tag "OnboardClock" ("Sample Clock Source"), "error in"=w375) -> ("task out"=w366:refnum<k21>, "error out"=w365:errorcluster)  [unwired: 8 in]
        n165 = local read "Audio sample rate (Hz)"() -> (w356:i64)
        n166 = local read "Pre-trigger time* (s)"() -> (w357:dbl)
        n167 = property class="DAQmx Timing"(reference=w366, error in=w365) -> (reference out=w363:refnum<k21>, error out=w362:errorcluster, "SampClk.Rate"=→"Acquire sample rate (Hz)":dbl)
        n168 = Increment(x=w357) -> (x+1=w358:dbl)
        n169 = call <vilib>:"DAQmx Start Task.vi"("task/channels in"=w363, "error in"=w362) -> ("task out"=w360:refnum<k21>, "error out"=w359:errorcluster)  [unwired: 12 in]
        n170 = Multiply(x=w356, y=w358) -> (x*y=w355:dbl)
        n171 = Round Toward +Infinity(x=w355) -> (ceil(x): smallest int >= x=w354:dbl)
        n172 = To Long Integer(number=w354) -> (32bit integer=→"Audio buffer size (frames)":i32)
        n173 = case shown="No Error" w359 {
          selector: w359 -> [w379 w387]
          tunnel: [w380 T2."Stopping"] -> w352
          tunnel: [w379 errorcluster {"status"=FALSE, "code"=0, "source"=""} ("error IO")] -> w351
          frame No Error {
            n174 = local read "STOP"() -> (w378:bool)
            n175 = case shown="True" w378 {
              tunnel: [T2."Capturing" T2."Stopping"] -> w380
              frame False {
              }
              frame True {
              }
            }
          }
          frame Error {
            n176 = call <vilib>:"Simple Error Handler.vi"("error in (no error)"=w387) -> ()  [unwired: 4 in, 5 out]
            n177 = local write "Settings"(T9."Video capture" ("Settings")) -> ()
            n178 = One Button Dialog(message="Error in audio\ncapture initialization.\nDisabling audio capture.") -> ()  [unwired: 1 in, 1 out]
            n179 = local write "Enable audio capture"(FALSE ("Enable audio capture")) -> ()
          }
        }
      }
      frame "Capturing" {
        n180 = local read "Samples per\nacquisition chunk"() -> (w398:i32)
        n181 = call-poly <vilib>:"DAQmx Read.vi"("task/channels in"=w406, "number of samples per channel"=w398, "error in"=w404) -> ("task out"=w405:refnum<k21>, "data"=w390:waveform(dbl), "error out"=w402:errorcluster)  [unwired: 10 in]
        "Unfiltered audio" <- w390
        n182 = Enqueue Element(queue=w403, element=w390, timeout in ms (-1)=0, error in (no error)=w402) -> (queue out=w400:refnum<queue>, error out=w393:errorcluster)  [unwired: 1 out]
        n183 = Unbundle By Name(w390) -> ("t0"=w389:timestamp)
        n184 = Get Queue Status(queue=w400, error in (no error)=w393) -> (error out=w392:errorcluster, # elements in queue=w399:i32)  [unwired: 1 in, 6 out]
        n185 = global write "Latest DAQmx timestamp.vi" "Latest DAQmx timestamp"(w389) -> ()
        n186 = local read "Trigger mode"() -> (w395:enum16{"Manual", "GPIO", "Audio"})
        n187 = flat-sequence {
          tunnel: w399 -> [w419]
          frame #0 {
            n188 = local read "Samples per\nacquisition chunk"() -> (w416:i32)
            n189 = local read "Audio sample rate (Hz)"() -> (w418:i64)
            n190 = local read "Audio buffer size (frames)"() -> (w415:i32)
            n191 = Multiply(x=w419, y=w416) -> (x*y=w417:i32)
            n192 = To Double Precision Float(number=w417) -> (double precision float=w420:dbl)
            n193 = Divide(x=w415, y=w418) -> (x/y=→"Audio buffer\nsize (s)":dbl)
            n194 = Divide(x=w420, y=w415) -> (x/y=w423:dbl)
            n195 = Multiply(x=w423, y=100.0) -> (x*y=→"Audio buffer":dbl)
          }
        }
        n196 = case shown="\"Audio\"" w395 {
          tunnel: w394 -> [_ _ w413]
          tunnel: w390 -> [_ _ w412]
          tunnel: w392 -> [w408 w409 w411]
          tunnel: [w408 w409 w410] -> w391
          frame "Manual", Default {
          }
          frame "GPIO" {
          }
          frame "Audio" {
            # "If trigger mode is audio, send efference copy of audio to processing loop"
            n197 = Enqueue Element(queue=w413, element=w412, error in (no error)=w411) -> (error out=w410:errorcluster)  [unwired: 1 in, 2 out]
          }
        }
        n198 = case shown="No Error" w391 {
          selector: w391 -> [w425 w436]
          tunnel: [w426 T2."Stopping"] -> w397
          tunnel: [w425 errorcluster {"status"=FALSE, "code"=0, "source"=""} ("error IO")] -> w396
          frame No Error {
            n199 = local read "STOP"() -> (w424:bool)
            n200 = case shown="True" w424 {
              tunnel: [w430 T2."Stopping"] -> w426
              frame False {
                n201 = local read "Enable audio capture"() -> (w429:bool)
                n202 = local read "Capture"() -> (w428:bool)
                n203 = And(x=w428, y=w429) -> (x .and. y?=w427:bool)
                n204 = case shown="True" w427 {
                  tunnel: [T2."Stopping" T2."Capturing"] -> w430
                  frame False {
                  }
                  frame True {
                  }
                }
              }
              frame True {
              }
            }
          }
          frame Error {
            n205 = call <vilib>:"Simple Error Handler.vi"("error in (no error)"=w436) -> ()  [unwired: 4 in, 5 out]
            n206 = One Button Dialog(message="Error in audio capture") -> ()  [unwired: 1 in, 1 out]
          }
        }
      }
      frame "Stopping" {
        n207 = call <vilib>:"DAQmx Stop Task.vi"("task/channels in"=w443, "error in"=w442) -> ("task out"=w444:refnum<k21>, "error out"=w445:errorcluster)  [unwired: 12 in]
        n208 = global write "Latest DAQmx timestamp.vi" "Latest DAQmx timestamp"(timestamp(0 s since 1904-01-01) ("Latest DAQmx timestamp")) -> ()
        n209 = call <vilib>:"DAQmx Clear Task.vi"("task in"=w444, "error in"=w445) -> ("error out"=w441:errorcluster)  [unwired: 13 in]
        n210 = case shown="No Error" w441 {
          selector: w441 -> [w449 w454]
          tunnel: [w449 errorcluster {"status"=FALSE, "code"=0, "source"=""} ("error out")] -> w440
          tunnel: [T2."Stopped" T2."Stopped"] -> w439
          frame No Error {
          }
          frame Error {
            w455 = T19 4 items=["no dialog", "OK message", "continue or stop message", "OK message + warnings", "continue/stop + warnings"] ("type of dialog (OK msg:1)")
            n211 = One Button Dialog(message="Error stopping audio capture loop") -> ()  [unwired: 1 in, 1 out]
            n212 = local write "Trigger mode"(enum16{"Manual", "GPIO", "Audio"}."Manual" ("Trigger mode")) -> ()
            n213 = call <vilib>:"Simple Error Handler.vi"("type of dialog (OK msg:1)"=w455, "error in (no error)"=w454) -> ()  [unwired: 3 in, 5 out]
          }
        }
      }
      frame "Stopped" {
        n214 = local read "STOP"() -> (w456:bool)
        n215 = case shown="True" w456 {
          tunnel: [w461 T2."Exiting"] -> w457
          frame False {
            n216 = local read "Enable audio capture"() -> (w463:bool)
            n217 = local read "Capture"() -> (w464:bool)
            n218 = And(x=w464, y=w463) -> (x .and. y?=w462:bool)
            n219 = case shown="False" w462 {
              tunnel: [T2."Stopped" T2."Initializing"] -> w461
              frame False {
              }
              frame True {
              }
            }
          }
          frame True {
          }
        }
      }
      frame "Exiting" {
        n220 = Release Queue(queue=w471, force destroy? (F)=TRUE, error in (no error)=w469) -> (error out=w468:errorcluster)  [unwired: 2 out]
      }
    }
    "Audio capture state" <- w350
  }
  n221 = while {
    shift-right: [w486] -> w10
    shift-left: w31 -> [w482]
    shift-right: [w484] -> _
    shift-left: _ -> [w485]
    shift-right: [w481] -> _
    shift-left: T2."Stopping" -> [w483]
    tunnel: w6 -> [w479]
    tunnel: w33 -> [w480]
    shift-right: [w477] -> _
    shift-left: 0 -> [w478]
    tunnel: [w475] -> w20
    stop <- w475 stop-if-true
    # "Camera Capture Process"
    n222 = case shown="\"Capturing\"" w483 {
      tunnel: w482 -> [w519 w557 w609 w642 w651]
      tunnel: [w491 w573 T10 refnum ("Session Out") w639 w656] -> w484
      tunnel: [w501 w555 w604 w636 w650] -> w486
      tunnel: w485 -> [_ w551 w610 w639 w656]
      tunnel: [FALSE FALSE FALSE FALSE TRUE] -> w475
      tunnel: [w500 w570 w603 w638 T2."Exiting"] -> w481
      tunnel: w480 -> [_ w567 _ _ w653]
      tunnel: w479 -> [w506 w556 _ _ _]
      tunnel: w478 -> [w508 w561 w605 w637 w654]
      tunnel: [w508 w560 w605 w637 w654] -> w477
      frame "Initializing", Default {
        n223 = flat-sequence {
          frame #0 {
            w525 = T22."Page Disabled & Grayed" ("Page Enabled State")
            n224 = property on="Trigger write to file" class="Bool"("DisabledEnum"=T21."Enabled" ("Disabled")) -> ()  [unwired: 2 in, 2 out]
            n225 = property on="Settings" class="TabCtl (strict)"() -> ("Pages"=w530:refnum<vi>[])  [unwired: 2 in, 2 out]
            n226 = Index Array(array=w530, index #1=0 ("index"), index #2=3 ("index")) -> (element #1=w528:refnum<vi>, element #2=w526:refnum<vi>)  [unwired: 1 in, 1 out]
            n227 = property class="Page"(reference=w528, "PageEnb"=w525) -> ()  [unwired: 1 in, 2 out]
            n228 = property class="Page"(reference=w526, "PageEnb"=w525) -> ()  [unwired: 1 in, 2 out]
          }
        }
        n229 = call <vilib>:"IMAQdx Open Camera.vi"("error in"=w519, "Session In"="Select camera") -> ("error out"=w507:errorcluster, "Session Out"=w516:T10)  [unwired: 1 in, 7 out]
        n230 = Increment(x="Pre-trigger time* (s)") -> (x+1=w493:dbl)
        n231 = Multiply(x="Frames Per Second", y=w493) -> (x*y=w514:dbl)
        n232 = control-ref of="Events and errors"() -> (w490:refnum<vi>)
        n233 = Round Toward +Infinity(x=w514) -> (ceil(x): smallest int >= x=w513:dbl)
        n234 = call "ConfigureCamera.vi"("Line name"="GPIO line", "error in (no error)"=w507, "Frames Per Second"="Frames Per Second", "Automatic frame rate"="OFF" ("ValueString"), "Refnum in"=w516) -> ("error out"=w488:errorcluster, "Refnum out"=w499:T10)  [unwired: 5 in]
        n235 = call "logError.vi"("Error to log"=w488, "Location"="Setting camera attributes", "Text reference"=w490) -> ("error out"=w487:errorcluster)  [unwired: 8 in]
        n236 = To Long Integer(number=w513) -> (32bit integer=→"Video buffer size (frames)":i32)
        n237 = call <vilib>:"IMAQdx Configure Grab.vi"("error in"=w487, "Session In"=w499) -> ("error out"=w504:errorcluster, "Session Out"=w520:T10)  [unwired: 8 out]
        n238 = call "getRecycledImagePointer.vi"("error in (no error)"=w504, "Recycled image pointer queue in"=w506) -> ("error out"=w503:errorcluster, "Image pointer"=w505:T12)  [unwired: 6 in, 2 out]
        n239 = call <vilib>:"IMAQdx Grab.vi"("error in"=w503, "Image In"=w505, "Session In"=w520) -> ("error out"=w492:errorcluster, "Image Out"=w509:T12, "Session Out"=w491:T10)  [unwired: 1 in, 5 out]
        "Current camera session reference" <- w491
        n240 = call <vilib>:"IMAQdx Enumerate Attributes.vi"("Visibility"=IMAQdx_Attribute_Visibility."Advanced", "Session In"=w491) -> ("Attribute Information Array"=w497:T8)  [unwired: 7 in, 2 out]
        "Attribute Information Array" <- w497
        n241 = call "IMAQ AVI2 Get Codec Names"("Image"=w509) -> ("Codec Names"=w502:string[])  [unwired: 9 in, 1 out]
        n242 = for {
          tunnel: w497 -> [w524] mode=indexing
          tunnel: [w522] -> w496 mode=indexing
          n243 = Unbundle By Name(w524) -> ("Attribute Name"=w523:string)  [unwired: 3 out]
          n244 = Concatenate Strings(w523, "\r") -> (w522:string)
        }
        n245 = property on="Video codec**" class="CmbBox"("Strings[]"=w502) -> ()  [unwired: 2 in, 2 out]
        n246 = case shown="Error" w492 {
          selector: w492 -> [w534 w537]
          tunnel: [w534 w538] -> w501
          tunnel: [w533 w539] -> w500
          frame No Error {
            # "Everything went well, begin capture"
            n247 = local read "STOP"() -> (w532:bool)
            n248 = case shown="True" w532 {
              tunnel: [T2."Capturing" T2."Stopping"] -> w533
              frame False {
              }
              frame True {
              }
            }
          }
          frame Error {
            # "Camera not found, go to stopped state"
            n249 = Unbundle By Name(w537) -> ("code"=w540:i32)
            n250 = case shown="-1074360311" w540 {
              tunnel: [T2."Stopping" T2."Stopping"] -> w539
              tunnel: w537 -> [w542 _]
              tunnel: [errorcluster {"status"=FALSE, "code"=0, "source"=""} ("error IO") errorcluster {"status"=FALSE, "code"=0, "source"=""} ("error IO")] -> w538
              frame 0, Default {
                # "Unexpected error"
                n251 = call <vilib>:"Simple Error Handler.vi"("error in (no error)"=w542) -> ()  [unwired: 4 in, 5 out]
              }
              frame -1074360311 {
                # "Camera not found error"
                n252 = local write "Settings"(T9."Video capture" ("Settings")) -> ()
                n253 = One Button Dialog(message="Camera not found!\nCheck that camera is\nconnected an the correct\ncamera is selected.") -> ()  [unwired: 1 in, 1 out]
              }
            }
          }
        }
        n254 = Concatenate Strings(w496) -> (→"concatenated string":string)
      }
      frame "Capturing" {
        # "Capture from camera ==> buffer"
        n255 = call "getRecycledImagePointer.vi"("error in (no error)"=w557, "Image ID"=w561, "Recycled image pointer queue in"=w556) -> ("error out"=w558:errorcluster, "Next image ID"=w560:i32, "Image pointer"=w559:T12)  [unwired: 5 in, 1 out]
        n256 = call <vilib>:"IMAQdx Grab.vi"("error in"=w558, "Wait for Next Buffer? (Yes)"=TRUE, "Image In"=w559, "Session In"=w551) -> ("error out"=w563:errorcluster, "Buffer Number Out"=w569:u32, "Image Out"=w568:T12, "Session Out"=w573:T10)  [unwired: 4 out]
        "Video input" <- w568
        n257 = call "getLatestDAQmxTimestamp.vi"() -> ("Timestamp"=w554:timestamp)  [unwired: 10 in, 1 out]
        n258 = Add(x=w554, y="Estimated camera latency (s)") -> (x+y=w549:timestamp)
        n259 = Bundle("Image Out"=w568, w549) -> (w552:cluster{"Image Out":T12, timestamp})  [unwired: 1 in]
        n260 = Enqueue Element(queue=w567, element=w552, timeout in ms (-1)=0, error in (no error)=w563) -> (queue out=w565:refnum<queue>, error out=w562:errorcluster)  [unwired: 1 out]
        n261 = call <vilib>:"Simple Error Handler.vi"("error in (no error)"=w562) -> ("error out"=w553:errorcluster)  [unwired: 4 in, 4 out]
        n262 = Get Queue Status(queue=w565, error in (no error)=w553) -> (error out=w550:errorcluster, # elements in queue=w566:i32)  [unwired: 1 in, 6 out]
        n263 = case shown="Error" w550 {
          selector: w550 -> [w585 w594]
          tunnel: [w586 w597] -> w570
          tunnel: [w585 w595] -> w555
          frame No Error {
            n264 = local read "STOP"() -> (w584:bool)
            n265 = case shown="True" w584 {
              tunnel: [w590 T2."Stopping"] -> w586
              frame False {
                n266 = local read "Enable video capture"() -> (w589:bool)
                n267 = local read "Capture"() -> (w588:bool)
                n268 = And(x=w589, y=w588) -> (x .and. y?=w587:bool)
                n269 = case shown="True" w587 {
                  tunnel: [T2."Stopping" T2."Capturing"] -> w590
                  frame False {
                  }
                  frame True {
                  }
                }
              }
              frame True {
              }
            }
          }
          frame Error {
            n270 = Unbundle By Name(w594) -> ("code"=w596:i32)
            n271 = case shown="0, Default" w596 {
              tunnel: [T2."Stopping"] -> w597
              tunnel: [errorcluster {"status"=FALSE, "code"=0, "source"=""} ("error out")] -> w595
              tunnel: w594 -> [w601]
              frame 0, Default {
                w600 = T19 4 items=["no dialog", "OK message", "continue or stop message", "OK message + warnings", "continue/stop + warnings"] ("type of dialog (OK msg:1)")
                # "Unexpected error"
                n272 = call <vilib>:"Simple Error Handler.vi"("type of dialog (OK msg:1)"=w600, "error in (no error)"=w601) -> ()  [unwired: 3 in, 5 out]
                n273 = One Button Dialog(message="Error during camera capture") -> ()  [unwired: 1 in, 1 out]
              }
            }
          }
        }
        n274 = flat-sequence {
          tunnel: w569 -> [w583]
          tunnel: w566 -> [w575]
          frame #0 {
            n275 = To Double Precision Float(number=w575) -> (double precision float=w578:dbl)
            n276 = call <vilib>:"Calculate Frames per Second.vi"("Buffer Number"=w583) -> ("Missed Frames"=→"Missed Frames":bool, "Acquired Frames/s"=w577:dbl)  [unwired: 8 in, 1 out]
            "Acquire framerate (fps)" <- w577
            n277 = local read "Video buffer size (frames)"() -> (w574:i32)
            n278 = Divide(x=w574, y=w577) -> (x/y=→"Video buffer\n size (s)":dbl)
            n279 = Divide(x=w578, y=w574) -> (x/y=w582:dbl)
            n280 = Multiply(x=w582, y=100.0) -> (x*y=→"Video buffer":dbl)
          }
        }
      }
      frame "Stopping" {
        n281 = flat-sequence {
          frame #0 {
            w629 = T22."Page Enabled" ("Page Enabled State")
            w632 = 0.0 ("Buffer % full")
            n282 = local write "Capture"(FALSE ("Capture")) -> ()
            n283 = local write "Video buffer"(w632) -> ()
            n284 = local write "Video buffer\n size (s)"(w632) -> ()
            n285 = local write "Acquire framerate (fps)"(w632) -> ()
            n286 = property on="Settings" class="TabCtl (strict)"() -> ("Pages"=w627:refnum<vi>[])  [unwired: 2 in, 2 out]
            n287 = Index Array(array=w627, index #1=0 ("index"), index #2=3 ("index")) -> (element #1=w628:refnum<vi>, element #2=w626:refnum<vi>)
            n288 = property class="Page"(reference=w628, "PageEnb"=w629) -> ()  [unwired: 1 in, 2 out]
            n289 = property class="Page"(reference=w626, "PageEnb"=w629) -> ()  [unwired: 1 in, 2 out]
            n290 = property on="Trigger write to file" class="Bool"("DisabledEnum"=T21."Disabled and Grayed Out" ("Disabled")) -> ()  [unwired: 2 in, 2 out]
          }
        }
        n291 = call <vilib>:"IMAQdx Close Camera.vi"("error in"=w609, "Session In"=w610) -> ("error out"=w606:errorcluster)  [unwired: 9 out]
        n292 = case shown="Error" w606 {
          selector: w606 -> [w611 w613]
          tunnel: [T2."Stopped" w616] -> w603
          tunnel: [w611 w614] -> w604
          frame No Error {
          }
          frame Error {
            n293 = Unbundle By Name(w613) -> ("code"=w615:i32)
            n294 = case shown="-1074360316" w615 {
              tunnel: [T2."Stopped" T2."Stopped" T2."Stopped"] -> w616
              tunnel: [errorcluster {"status"=FALSE, "code"=0, "source"=""} ("error out") errorcluster {"status"=FALSE, "code"=0, "source"=""} ("error out") errorcluster {"status"=FALSE, "code"=0, "source"=""} ("error out")] -> w614
              tunnel: w613 -> [w620 _ _]
              frame 0, Default {
                w619 = T19 4 items=["no dialog", "OK message", "continue or stop message", "OK message + warnings", "continue/stop + warnings"] ("type of dialog (OK msg:1)")
                # "Unexpected error"
                n295 = call <vilib>:"Simple Error Handler.vi"("type of dialog (OK msg:1)"=w619, "error in (no error)"=w620) -> ()  [unwired: 3 in, 5 out]
                n296 = One Button Dialog(message="Error while stopping camera capture") -> ()  [unwired: 1 in, 1 out]
              }
              frame -1074360306 {
                # "No acquisition to close, ignore error"
              }
              frame -1074360316 {
                # "No acquisition to close, ignore error"
              }
            }
          }
        }
      }
      frame "Stopped" {
        # "Do not capture from camera ==> buffer"
        n297 = Wait (ms)(milliseconds to wait=u32 100) -> ()  [unwired: 1 out]
        n298 = call <vilib>:"Clear Errors.vi"("error in (no error)"=w642) -> ("error out"=w636:errorcluster)  [unwired: 5 in, 1 out]
        n299 = local read "STOP"() -> (w635:bool)
        n300 = case shown="True" w635 {
          tunnel: [w646 T2."Exiting"] -> w638
          frame False {
            n301 = And(x="Capture", y="Enable video capture") -> (x .and. y?=w643:bool)
            n302 = case shown="True" w643 {
              tunnel: [T2."Stopped" T2."Initializing"] -> w646
              frame False {
              }
              frame True {
              }
            }
          }
          frame True {
          }
        }
      }
      frame "Exiting" {
        (unwired) refnum<queue> refnum ("queue out")
        n303 = Release Queue(queue=w653, force destroy? (F)=TRUE, error in (no error)=w651) -> (error out=w650:errorcluster)  [unwired: 2 out]
      }
    }
    n304 = Wait (ms)(milliseconds to wait=u32 0) -> ()  [unwired: 1 out]
    "Video capture state" <- w483
  }
  n305 = while {
    shift-right: [w679] -> w9
    shift-left: _ -> [w678]
    shift-right: [w675] -> _
    shift-left: T1."Stopped" -> [w677]
    shift-right: [w674] -> _
    shift-left: _ -> [w673]
    tunnel: w6 -> [w672]
    tunnel: w29 -> [w671]
    tunnel: w33 -> [w676]
    tunnel: w2 -> [w670]
    shift-right: [w669] -> _
    shift-left: _ -> [w668]
    tunnel: [w666] -> w15
    shift-right: [w665] -> _
    shift-left: _ -> [w661]
    shift-right: [w664] -> _
    shift-left: _ -> [w662]
    tunnel: w7 -> [w663]
    tunnel: w6 -> [w660]
    shift-right: [w658] -> _
    shift-left: T5 [] -> [w659]
    stop <- w666 stop-if-true
    # "File writing Process"
    n306 = Wait (ms)(milliseconds to wait=u32 0) -> ()  [unwired: 1 out]
    n307 = case shown="\"Stopped\"" w677 {
      tunnel: [w703 w784 w856 w912 w976] -> w679
      tunnel: [w705 w787 T23 refnum ("AVI Refnum (duplicate)") w915 w980] -> w674
      tunnel: w678 -> [w689 w768 w866 w900 w977]
      tunnel: [w707 w788 w855 w917 T1."Exiting"] -> w675
      tunnel: [FALSE FALSE FALSE FALSE TRUE] -> w666
      tunnel: w676 -> [w686 w789 _ w901 _]
      tunnel: w673 -> [_ w786 w865 w915 w980]
      tunnel: w672 -> [w685 w785 _ _ w975]
      tunnel: w671 -> [_ w771 _ w914 _]
      tunnel: w670 -> [_ _ w861 _ _]
      tunnel: [w702 w782 w859 w911 w979] -> w669
      tunnel: w668 -> [_ w782 w859 w911 w979]
      tunnel: [w701 w780 w854 w909 w974] -> w665
      tunnel: [w700 w779 T24 refnum ("sound file refnum out") w910 w973] -> w664
      tunnel: w663 -> [w687 w763 _ w907 _]
      tunnel: w662 -> [_ w781 w851 w910 w973]
      tunnel: w661 -> [_ w780 w854 w909 w974]
      tunnel: w660 -> [_ _ _ w904 _]
      tunnel: w659 -> [w695 w772 w848 w898 w972]
      tunnel: [w695 w765 w848 w895 w972] -> w658
      frame "Initializing", Default {
        n308 = local read "Samples per\nacquisition chunk"() -> (w683:i32)
        n309 = local read "Audio sample rate (Hz)"() -> (w684:i64)
        n310 = Index Array(array=w695, index=0) -> (element=w694:T4)
        n311 = Unbundle By Name(w694) -> ("Trigger time"=w697:timestamp)
        n312 = To Double Precision Float(number=w683) -> (double precision float=w681:dbl)
        n313 = To Double Precision Float(number=w684) -> (double precision float=w682:dbl)
        n314 = Divide(x=w681, y=w682) -> (x/y=w680:dbl)
        n315 = call "alignAudioVideoQueues.vi"("Image pointer recycling queue"=w685, "error in (no error)"=w689, "Alignment tolerance"=w680, "Video queue in"=w686, "Audio queue in"=w687) -> ("error out"=w688:errorcluster)  [unwired: 3 in, 3 out]
        n316 = local read "Enable audio write"() -> (w691:bool)
        n317 = local read "Enable video write"() -> (w690:bool)
        n318 = case shown="True" w691 {
          tunnel: "Write directory" -> [_ w747]
          tunnel: "Base Filename (no extension)" -> [_ w745]
          tunnel: [path "" ("Available file path") w734] -> w701
          tunnel: [T24 refnum ("sound file refnum") w743] -> w700
          tunnel: [w730 w732] -> w698
          tunnel: w697 -> [_ w741]
          tunnel: w688 -> [w730 w739]
          frame False {
          }
          frame True {
            # "Initialize audio file"
            n319 = Concatenate Strings(w745, ".wav" ("Audio extension")) -> (w740:string)
            n320 = local read "Audio sample rate (Hz)"() -> (w738:i64)
            n321 = call "createUsableFilename.vi"("error in (no error)"=w739, "Timestamp"=w741, "Base filename"=w740, "Write directory"=w747) -> ("error out"=w742:errorcluster, "Available file path"=w734:path)  [unwired: 6 in]
            n322 = Bundle By Name(cluster=T25 {"sample rate (S/s)"=22050.0, "number of channels"=2, "bits per sample"=16} ("sound format"), "sample rate (S/s)"=w738, "number of channels"=1, "bits per sample"="bits per sample") -> (w746:T25)
            n323 = call-poly <vilib>:"Sound File Open.vi"("error in (no error)"=w742, "sound format"=w746, "path"=w734) -> ("error out"=w733:errorcluster, "sound file refnum"=w743:T24)  [unwired: 7 in]
            n324 = Path To String(path=w734) -> (string=w735:string)
            n325 = control-ref of="Events and errors"() -> (w737:refnum<vi>)
            n326 = Concatenate Strings("Audio file write initializing: " ("New log entry"), w735) -> (w736:string)
            n327 = call "logEvent.vi"("error in (no error)"=w733, "New log entry"=w736, "Text reference"=w737) -> ("error out"=w732:errorcluster)  [unwired: 8 in]
          }
        }
        n328 = case shown="True" w690 {
          tunnel: [T23 refnum ("AVI Refnum") w727] -> w705
          tunnel: [w710 w711] -> w704
          tunnel: [path "" ("Available file path") w713] -> w702
          tunnel: "Write directory" -> [_ w722]
          tunnel: "Base Filename (no extension)" -> [_ w721]
          tunnel: w697 -> [_ w720]
          tunnel: w688 -> [w710 w718]
          frame False {
          }
          frame True {
            # "Initialize video file"
            n329 = Concatenate Strings(w721, ".avi" ("Video extension")) -> (w719:string)
            n330 = call "createUsableFilename.vi"("error in (no error)"=w718, "Timestamp"=w720, "Base filename"=w719, "Write directory"=w722) -> ("error out"=w726:errorcluster, "Available file path"=w713:path)  [unwired: 6 in]
            n331 = call "IMAQ AVI2 Create"("error in (no error)"=w726, "Codec"="Video codec**", "Frames Per Second"=u32 30, "AVI Path"=w713) -> ("error out"=w712:errorcluster, "AVI Refnum"=w727:T23)  [unwired: 6 in]
            n332 = Path To String(path=w713) -> (string=w717:string)
            n333 = control-ref of="Events and errors"() -> (w715:refnum<vi>)
            n334 = Concatenate Strings("Video file write initializing: " ("New log entry"), w717) -> (w716:string)
            n335 = call "logEvent.vi"("error in (no error)"=w712, "New log entry"=w716, "Text reference"=w715) -> ("error out"=w711:errorcluster)  [unwired: 8 in]
          }
        }
        n336 = flat-sequence {
          frame #0 {
            # "Disable/enable controls"
            n337 = property on="Settings" class="TabCtl (strict)"() -> ("Pages"=w751:refnum<vi>[])  [unwired: 2 in, 2 out]
            n338 = Index Array(array=w751, index=1) -> (element=w753:refnum<vi>)
            n339 = property class="Page"(reference=w753, "PageEnb"=T22."Page Disabled & Grayed" ("Page Enabled State")) -> ()  [unwired: 1 in, 2 out]
          }
        }
        n340 = Merge Errors(w704, w698) -> (w699:errorcluster)
        n341 = case shown="Error" w699 {
          selector: w699 -> [w755 w760]
          tunnel: [T1."Saving" T1."Closing file"] -> w707
          tunnel: [w755 w757] -> w703
          frame No Error {
          }
          frame Error {
            n342 = control-ref of="Events and errors"() -> (w759:refnum<vi>)
            n343 = call "logError.vi"("Error to log"=w760, "Location"="File write init", "Text reference"=w759) -> ("error out"=w757:errorcluster)  [unwired: 8 in]
            n344 = local write "Settings"(T9."File writing" ("Settings")) -> ()
          }
        }
      }
      frame "Saving" {
        # "Write frames from buffer ==> file."
        n345 = call "updateTriggerList.vi"("error in (no error)"=w768, "Trigger list"=w772, "Trigger queue in"=w771) -> ("error out"=w770:errorcluster, "Updated trigger list"=w764:T5)  [unwired: 5 in, 2 out]
        n346 = local read "Enable video write"() -> (w774:bool)
        n347 = local write "Updated trigger list"(w764) -> ()
        n348 = local read "Enable audio write"() -> (w773:bool)
        n349 = Index Array(array=w764, index=0) -> (element=w767:T4)
        "Current video trigger times" <- w767
        n350 = case shown="False" w774 {
          tunnel: w789 -> [w810 w819]
          tunnel: [w805 w818] -> w787
          tunnel: w786 -> [w805 w817]
          tunnel: w785 -> [w809 w816]
          tunnel: [w807 w815] -> w783
          tunnel: w767 -> [_ w814]
          tunnel: [FALSE ("Writing video?") w813] -> w778
          tunnel: w770 -> [w808 w812]
          frame False {
            # "Video write not enabled. Instead, maintain size of video buffer"
            n351 = local read "Video buffer size (frames)"() -> (w811:i32)
            n352 = call "maintainVideoBuffer.vi"("error in (no error)"=w808, "Video buffer size (frames)"=w811, "Image pointer recycling queue"=w809, "Video queue"=w810) -> ("error out"=w807:errorcluster)  [unwired: 7 in]
          }
          frame True {
            # "Video write enabled - write video!"
            n353 = call "writeVideo.vi"("Image pointer recycler queue"=w816, "error in (no error)"=w812, "Trigger timestamps"=w814, "Video queue"=w819, "AVI file reference in"=w817) -> ("error out"=w815:errorcluster, "Writing video?"=w813:bool, "AVI file reference out"=w818:T23)  [unwired: 3 in, 1 out]
          }
        }
        "Writing video" <- w778
        n354 = case shown="False" w773 {
          tunnel: w763 -> [w792 w804]
          tunnel: w781 -> [w791 w803]
          tunnel: [w791 w802] -> w779
          tunnel: w767 -> [_ w801]
          tunnel: [FALSE ("Writing audio?") w800] -> w777
          tunnel: w770 -> [w794 w799]
          tunnel: [w793 w798] -> w775
          frame False {
            # "Audio write not enabled. Instead, maintain buffer size"
            n355 = local read "Samples per\nacquisition chunk"() -> (w796:i32)
            n356 = local read "Audio buffer size (frames)"() -> (w795:i32)
            n357 = call "maintainAudioBuffer.vi"("error in (no error)"=w794, "Samples per\nacquisition chunk"=w796, "Audio buffer size (frames)"=w795, "Audio data queue in"=w792) -> ("error out"=w793:errorcluster)  [unwired: 7 in]
          }
          frame True {
            # "Audio write enabled - write audio!"
            n358 = call "writeAudio.vi"("error in (no error)"=w799, "WAV file reference in"=w803, "Trigger timestamps"=w801, "Queue in"=w804) -> ("error out"=w798:errorcluster, "Writing audio?"=w800:bool, "WAV file reference out"=w802:T24)  [unwired: 4 in, 1 out]
          }
        }
        "Writing audio" <- w777
        n359 = Or(x=w778, y=w777) -> (x .or. y?=w766:bool)
        n360 = Merge Errors(w783, w775) -> (w776:errorcluster)
        n361 = case shown="Error" w776 {
          selector: w776 -> [w823 w839]
          tunnel: [w825 T1."Closing file"] -> w788
          tunnel: [w823 errorcluster {"status"=FALSE, "code"=0, "source"=""} ("error IO")] -> w784
          tunnel: w766 -> [w824 _]
          tunnel: w764 -> [w821 w842]
          tunnel: [w820 w842] -> w765
          frame No Error {
            n362 = local read "STOP"() -> (w822:bool)
            n363 = case shown="False" w822 {
              tunnel: [w829 T1."Closing file"] -> w825
              tunnel: w824 -> [w828 _]
              tunnel: w821 -> [w827 w837]
              tunnel: [w826 w837] -> w820
              frame False {
                # "Stop signal not received"
                n364 = case shown="False" w828 {
                  tunnel: [T1."Closing file" T1."Saving"] -> w829
                  tunnel: w827 -> [w831 w835]
                  tunnel: [w830 w835] -> w826
                  frame False {
                    # "Done saving, remove trigger from list, close files."
                    n365 = Delete From Array(array=w831, length=1, index=0) -> (array with subset deleted=w830:T5)  [unwired: 1 out]
                  }
                  frame True {
                    # "Not done saving"
                  }
                }
              }
              frame True {
                # "Stop signal received - exit loop"
              }
            }
          }
          frame Error {
            n366 = control-ref of="Events and errors"() -> (w840:refnum<vi>)
            n367 = call "logError.vi"("Error to log"=w839, "Location"="File write saving", "Text reference"=w840) -> ()  [unwired: 8 in, 1 out]
          }
        }
      }
      frame "Closing file" {
        n368 = flat-sequence {
          frame #0 {
            n369 = property on="Settings" class="TabCtl (strict)"() -> ("Pages"=w892:refnum<vi>[])  [unwired: 2 in, 2 out]
            n370 = Index Array(array=w892, index=1) -> (element=w893:refnum<vi>)
            n371 = property class="Page"(reference=w893, "PageEnb"=T22."Page Enabled" ("Page Enabled State")) -> ()  [unwired: 1 in, 2 out]
          }
        }
        n372 = call "IMAQ AVI2 Close"("error in (no error)"=w866, "AVI Refnum"=w865) -> ("error out"=w853:errorcluster)  [unwired: 9 in]
        "Error after closing AVI" <- w853
        n373 = local write "Writing video"(FALSE ("Writing video")) -> ()
        n374 = local write "Writing audio"(FALSE ("Writing audio")) -> ()
        n375 = call <vilib>:"Sound File Close.vi"("error in (no error)"=w853, "sound file refnum"=w851) -> ("error out"=w852:errorcluster)  [unwired: 9 in]
        "Error after closing WAV" <- w852
        n376 = local read "Enable audio write"() -> (w858:bool)
        n377 = local read "Enable audio write"() -> (w847:bool)
        n378 = Compound Arithmetic op=AND("Combine audio & \nvideo into one file*", w858, w847) -> (w860:bool)
        n379 = case shown="True" w860 {
          tunnel: w852 -> [w875 w883]
          tunnel: [w875 w879] -> w857
          tunnel: w861 -> [_ w885]
          tunnel: w859 -> [_ w884]
          tunnel: w854 -> [_ w881]
          frame False {
            # "Don't mux audio and video"
          }
          frame True {
            # "Send video file path to the muxing loop to be muxed"
            n380 = Bundle(cluster=T13 {"Video path"=path "", "Audio path"=path ""}, "Video path"=w884, "Audio path"=w881) -> (w880:T13)
            "mux path cluster" <- w880
            n381 = Enqueue Element(queue=w885, element=w880, timeout in ms (-1)=10, error in (no error)=w883) -> (timed out?=w878:bool, error out=w882:errorcluster)  [unwired: 1 out]
            "Error after sending paths to mux loop" <- w882
            n382 = case shown="True" w878 {
              tunnel: w882 -> [w886 w890]
              tunnel: [w886 w889] -> w879
              frame False {
              }
              frame True {
                n383 = call <vilib>:"Error Cluster From Error Code.vi"("error in (no error)"=w890, "error message (\"\")"="Could not enqueue path\n element to mux loop" ("error message (\"\")"), "error code (0)"=-772277) -> ("error out"=w889:errorcluster)  [unwired: 6 in]
              }
            }
          }
        }
        n384 = control-ref of="Events and errors"() -> (w845:refnum<vi>)
        n385 = call "logEvent.vi"("New log entry"="File writing closing", "Text reference"=w845) -> ()  [unwired: 9 in, 1 out]
        n386 = case shown="Error" w857 {
          selector: w857 -> [w868 w870]
          tunnel: [w868 errorcluster {"status"=FALSE, "code"=0, "source"=""} ("error IO")] -> w856
          tunnel: [T1."Stopped" T1."Stopped"] -> w855
          frame No Error {
          }
          frame Error {
            n387 = control-ref of="Events and errors"() -> (w871:refnum<vi>)
            n388 = call "logError.vi"("Error to log"=w870, "Location"="File write closing", "Text reference"=w871) -> ()  [unwired: 8 in, 1 out]
          }
        }
      }
      frame "Stopped" {
        # "Do not capture frames from buffer ==> file. Maintain size of buffers by discarding overflowing data."
        n389 = local read "Video buffer size (frames)"() -> (w905:i32)
        n390 = local read "Samples per\nacquisition chunk"() -> (w906:i32)
        n391 = local read "Audio buffer size (frames)"() -> (w899:i32)
        n392 = call "maintainVideoBuffer.vi"("error in (no error)"=w900, "Video buffer size (frames)"=w905, "Image pointer recycling queue"=w904, "Video queue"=w901) -> ("error out"=w902:errorcluster)  [unwired: 7 in]
        n393 = call "maintainAudioBuffer.vi"("error in (no error)"=w900, "Samples per\nacquisition chunk"=w906, "Audio buffer size (frames)"=w899, "Audio data queue in"=w907) -> ("error out"=w908:errorcluster)  [unwired: 7 in]
        n394 = Merge Errors(w908, w902) -> (w903:errorcluster)
        n395 = call "updateTriggerList.vi"("error in (no error)"=w903, "Trigger list"=w898, "Trigger queue in"=w914) -> ("error out"=w913:errorcluster, "Trigger available?"=w897:bool, "Updated trigger list"=w896:T5)  [unwired: 5 in, 1 out]
        n396 = case shown="No Error" w913 {
          selector: w913 -> [w922 w967]
          tunnel: [w923 T1."Stopped"] -> w917
          tunnel: [w922 w966] -> w912
          tunnel: w897 -> [w920 _]
          tunnel: w896 -> [w919 w970]
          tunnel: [w918 w970] -> w895
          frame No Error {
            n397 = local read "STOP"() -> (w921:bool)
            n398 = case shown="False" w921 {
              tunnel: [w927 T1."Exiting"] -> w923
              tunnel: w920 -> [w926 _]
              tunnel: w919 -> [w925 w964]
              tunnel: [w924 w964] -> w918
              frame False {
                n399 = case shown="True" w926 {
                  tunnel: [T1."Stopped" w937] -> w927
                  tunnel: w925 -> [w928 w934]
                  tunnel: [w928 w933] -> w924
                  frame False {
                    # "No trigger, don't start"
                  }
                  frame True {
                    # "Trigger available!"
                    n400 = Index Array(array=w934) -> (element=w935:T4)  [unwired: 1 in]
                    n401 = Get Date/Time In Seconds() -> (seconds since 1Jan1904=w936:timestamp)
                    n402 = call "timestampInRange.vi"("Time Stamp"=w936, "Start and end times"=w935) -> ("timeState"=w932:T17)  [unwired: 9 in]
                    n403 = Not Equal?(x=w932, y=T17."At or after end") -> (x != y?=w930:bool)
                    n404 = case shown="True" w930 {
                      tunnel: [T1."Stopped" w953] -> w937
                      tunnel: w934 -> [w941 w944]
                      tunnel: [w940 w943] -> w933
                      frame False {
                        # "Trigger is expired. Remove it and do nothing."
                        n405 = Delete From Array(array=w941, length=1, index=0) -> (array with subset deleted=w940:T5)  [unwired: 1 out]
                      }
                      frame True {
                        # "Trigger is fresh! Act on it."
                        n406 = local read "Base Filename (no extension)"() -> (w950:string)
                        n407 = local read "Write directory"() -> (w948:path)
                        n408 = Path To String(path=w948) -> (string=w949:string)
                        n409 = String Length(string=w950) -> (length=w951:i32)
                        n410 = String Length(string=w949) -> (length=w952:i32)
                        n411 = Greater Than 0?(x=w951) -> (x > 0?=w947:bool)
                        n412 = Greater Than 0?(x=w952) -> (x > 0?=w946:bool)
                        n413 = And(x=w947, y=w946) -> (x .and. y?=w945:bool)
                        n414 = case shown="False" w945 {
                          tunnel: [T1."Stopped" T1."Initializing"] -> w953
                          tunnel: w944 -> [w958 w962]
                          tunnel: [w957 w962] -> w943
                          frame False {
                            # "No file path entered"
                            n415 = Delete From Array(array=w958, length=1, index=0) -> (array with subset deleted=w957:T5)  [unwired: 1 out]
                            n416 = local write "Settings"(T9."File writing" ("Settings")) -> ()
                            n417 = control-ref of="Events and errors"() -> (w956:refnum<vi>)
                            n418 = call "logEvent.vi"("New log entry"="ERROR: Write directory path blank. Ignoring trigger. Please enter a directory to save in and a filename.", "Text reference"=w956) -> ()  [unwired: 9 in, 1 out]
                          }
                          frame True {
                            # "File path has been entered."
                          }
                        }
                      }
                    }
                  }
                }
              }
              frame True {
              }
            }
          }
          frame Error {
            n419 = control-ref of="Events and errors"() -> (w968:refnum<vi>)
            n420 = call "logError.vi"("Error to log"=w967, "Location"="File write init", "Text reference"=w968) -> ("error out"=w966:errorcluster)  [unwired: 8 in]
            "detecting write trigger signal" <- w967
          }
        }
        "Updated trigger list" <- w898
      }
      frame "Exiting" {
        n421 = Release Queue(queue=w975, force destroy? (F)=TRUE, error in (no error)=w977) -> (error out=w976:errorcluster)  [unwired: 2 out]
      }
    }
    "Write state" <- w677
  }
  n422 = call "generateInitialTriggerTimes.vi"() -> ("Trigger message"=w5:T15)  [unwired: 11 in]
  n423 = while {
    tunnel: w29 -> [w1006]
    shift-right: [w987] -> _
    shift-left: w5 -> [w1004]
    shift-right: [w1000] -> w12
    shift-left: _ -> [w1003]
    tunnel: w28 -> [w1002]
    tunnel: w26 -> [w999]
    shift-right: [w996] -> _
    shift-left: w25 -> [w997]
    shift-right: [w995] -> _
    shift-left: w24 -> [w998]
    shift-right: [w993] -> _
    shift-left: w23 -> [w994]
    tunnel: [w988] -> w18
    stop <- w988 stop-if-true
    # "Trigger detection loop"
    n424 = Unbundle By Name(w1004) -> ("Trigger timestamps"=w985:T4)
    n425 = Get Date/Time In Seconds() -> (seconds since 1Jan1904=w983:timestamp)
    n426 = Tick Count (ms)() -> (millisecond timer value=w990:u32)
    n427 = call "timestampInRange.vi"("Time Stamp"=w983, "Start and end times"=w985) -> ("timeState"=w984:T17)  [unwired: 9 in]
    n428 = feedback-in #1(w990) -> ()
    n429 = feedback #1() -> (w991:u32)  [unwired: 1 in]
    n430 = Subtract(x=w990, y=w991) -> (x-y=→"dt audio trigger loop":u32)
    n431 = case shown="\"Audio\"" "Trigger mode" {
      tunnel: ["Trigger write to file" w1056 w1078] -> w993
      tunnel: w1004 -> [_ _ w1076]
      tunnel: [w1039 w1054 w1091] -> w1001
      tunnel: w1003 -> [w1039 w1055 w1087]
      tunnel: w1002 -> [_ _ w1092]
      tunnel: w998 -> [_ _ w1084]
      tunnel: w997 -> [_ _ w1085]
      tunnel: [w1038 w1050 w1082] -> w996
      tunnel: [w1038 w1050 w1081] -> w995
      tunnel: w994 -> [_ w1049 _]
      tunnel: [u32 10 ("milliseconds to wait") u32 0 ("milliseconds to wait") u32 0 ("milliseconds to wait")] -> w992
      tunnel: [w1031 w1042 w1077] -> w986
      tunnel: w984 -> [_ _ w1075]
      tunnel: w983 -> [w1030 w1041 w1074]
      frame "Manual", Default {
        w1038 = bool[] [] ("High threshold buffer")
        n432 = local read "Pre-trigger time* (s)"() -> (w1035:dbl)
        n433 = local read "Record length* (s)"() -> (w1036:dbl)
        n434 = call "calculateTriggerTimes.vi"("Current time"=w1030, "Record length* (s)"=w1036, "Pre-trigger time* (s)"=w1035) -> ("Trigger timestamps"=w1033:T4)  [unwired: 8 in]
        n435 = Bundle By Name(cluster=T15 {"Trigger timestamps"={"Start time"=timestamp(0 s since 1904-01-01), "Trigger time"=timestamp(0 s since 1904-01-01), "End time"=timestamp(0 s since 1904-01-01)}, "Message type"=enum."New trigger"} ("Trigger message"), "Trigger timestamps"=w1033, "Message type"=Trigger_message."New trigger") -> (w1031:T15)
      }
      frame "GPIO" {
        (unwired) FALSE
        w1050 = bool[] [] ("High threshold buffer")
        n436 = local read "Video capture state"() -> (w1053:T2)
        n437 = Equal?(x=w1053, y=T2."Capturing" ("Video capture state")) -> (x = y?=w1051:bool)
        n438 = case shown="True" w1051 {
          tunnel: [FALSE ("ValueBool") w1061] -> w1056
          tunnel: w1055 -> [w1058 w1064]
          tunnel: [w1058 w1062] -> w1054
          tunnel: w1049 -> [_ w1060]
          frame False {
            # "Capture hasn't begun yet, so camera session won't be valid yet."
          }
          frame True {
            n439 = Not(x=w1060) -> (.not. x?=w1059:bool)
            n440 = local read "Current camera session reference"() -> (w1067:T10)
            n441 = property class="IMAQdx"(reference=w1067, error in=w1064, "ActiveAttribute"="CameraAttributes::DigitalIOControl::LineStatus") -> (error out=w1063:errorcluster, "ValueBool"=w1065:bool)  [unwired: 1 out]
            n442 = And(x=w1065, y=w1059) -> (x .and. y?=w1061:bool)
            n443 = case shown="No Error" w1063 {
              selector: w1063 -> [w1068 w1069]
              tunnel: [w1068 errorcluster {"status"=FALSE, "code"=0, "source"=""} ("error IO")] -> w1062
              frame No Error {
              }
              frame Error {
                n444 = call <vilib>:"Simple Error Handler.vi"("error in (no error)"=w1069) -> ()  [unwired: 4 in, 5 out]
                n445 = local write "Trigger mode"(enum16{"Manual", "GPIO", "Audio"}."Manual" ("Trigger mode")) -> ()
                n446 = One Button Dialog(message="Error polling GPIO trigger line") -> ()  [unwired: 1 in, 1 out]
              }
            }
          }
        }
        n447 = local read "Pre-trigger time* (s)"() -> (w1046:dbl)
        n448 = local read "Record length* (s)"() -> (w1047:dbl)
        n449 = call "calculateTriggerTimes.vi"("Current time"=w1041, "Record length* (s)"=w1047, "Pre-trigger time* (s)"=w1046) -> ("Trigger timestamps"=w1044:T4)  [unwired: 8 in]
        n450 = Bundle By Name(cluster=T15 {"Trigger timestamps"={"Start time"=timestamp(0 s since 1904-01-01), "Trigger time"=timestamp(0 s since 1904-01-01), "End time"=timestamp(0 s since 1904-01-01)}, "Message type"=enum."New trigger"} ("Trigger message"), "Trigger timestamps"=w1044, "Message type"=Trigger_message."New trigger") -> (w1042:T15)
      }
      frame "Audio" {
        # "Measure filtered audio amplitude and calculate % of time audio has remained above high volume threshold and below low volume threshold for given periods of time. If it meets the criteria, signal loops to start or stop saving."
        n451 = Dequeue Element(queue=w1092, timeout in ms (-1)=0, error in (no error)=w1087) -> (element=w1090:waveform(dbl), timed out?=w1079:bool, error out=w1086:errorcluster)  [unwired: 1 out]
        n452 = case shown="False" w1079 {
          tunnel: w1090 -> [w1113 _]
          tunnel: [w1112 FALSE ("Mean under low threshold for required %")] -> w1089
          tunnel: [w1111 FALSE ("Boolean")] -> w1088
          tunnel: w1085 -> [w1110 w1117]
          tunnel: w1084 -> [w1109 w1116]
          tunnel: [w1108 w1117] -> w1082
          tunnel: [w1107 w1116] -> w1081
          frame False {
            # "Audio data received"
            n453 = local read "Samples per\nacquisition chunk"() -> (w1101:i32)
            n454 = call "CalculateAudioTriggerState.vi"("Low cutoff freq (Hz)"="Low cutoff freq (Hz)", "element"=w1113, "Audio sample rate (Hz)"="Audio sample rate (Hz)", "Low buffer in"=w1109, "High Audio Threshold"="High Audio Threshold", "Low Audio Threshold"="Low Audio Threshold", "Low monitoring period (s)"="Low monitoring period (s)", "High cutoff freq (Hz)"="High cutoff freq (Hz)", "Samples per\nacquisition chunk"=w1101, "High buffer in"=w1110, "Low Audio Threshold %"="Low Audio Threshold %", "High Audio Threshold %"="High Audio Threshold %", "High monitoring period (s)"="High monitoring period (s)") -> ("Mean above high threshold for required %"=w1111:bool, "Updated high buffer out"=w1108:bool[], "Updated low buffer out"=w1107:bool[], "Mean under low threshold for required %"=w1112:bool, "% of period above high threshold"=→"% above high threshold":dbl, "% of period below low threshold"=→"% below low threshold":dbl, "Filtered audio amplitude"=→"Filtered audio amplitude":T11, "Filtered audio"=→"Filtered audio":waveform(dbl))  [unwired: 7 in]
            "Mean under low threshold for required %" <- w1112
            "Mean above high threshold for required %" <- w1111
          }
          frame True {
            # "No audio data received"
          }
        }
        n455 = case shown="Error" w1086 {
          selector: w1086 -> [w1118 w1121]
          tunnel: [w1118 errorcluster {"status"=FALSE, "code"=0, "source"=""} ("error IO")] -> w1091
          frame No Error {
          }
          frame Error {
            n456 = call <vilib>:"Simple Error Handler.vi"("error in (no error)"=w1121) -> ()  [unwired: 4 in, 5 out]
            n457 = One Button Dialog(message="Audio trigger error") -> ()  [unwired: 1 in, 1 out]
          }
        }
        n458 = case shown="\"At or before start\", Default" w1075 {
          tunnel: w1076 -> [w1131 w1152]
          tunnel: w1089 -> [w1123 w1151]
          tunnel: w1088 -> [w1133 w1145]
          tunnel: [w1132 w1150] -> w1078
          tunnel: [w1126 w1149] -> w1077
          tunnel: w1074 -> [w1125 w1148]
          tunnel: "Audio trigger enable" -> [w1124 w1146]
          frame "At or before start", Default {
            # "We are not currently in a trigger time period."
            n459 = Not(x=w1123) -> (.not. x?=w1122:bool)
            n460 = Compound Arithmetic op=AND(w1124, w1133, w1122) -> (w1130:bool)
            n461 = case shown="True" w1130 {
              tunnel: [w1135 w1139] -> w1128
              tunnel: [FALSE ("Mean above high threshold?") TRUE ("Mean above high threshold?")] -> w1132
              tunnel: w1131 -> [w1136 _]
              tunnel: [Trigger_message."New trigger" ("Message type") Trigger_message."New trigger" ("Message type")] -> w1127
              tunnel: w1125 -> [_ w1138]
              frame False {
                # "Do not start new trigger period"
                n462 = Unbundle By Name(w1136) -> ("Trigger timestamps"=w1135:T4)
              }
              frame True {
                # "Audio averages above high threshold long enough (& not below low thresh)\nStart trigger period!"
                n463 = local read "Pre-trigger time* (s)"() -> (w1142:dbl)
                n464 = call "calculateTriggerTimes.vi"("Current time"=w1138, "Record length* (s)"="Time cutoff (s)", "Pre-trigger time* (s)"=w1142) -> ("Trigger timestamps"=w1139:T4)  [unwired: 8 in]
              }
            }
            n465 = Bundle By Name(cluster=T15 {"Trigger timestamps"={"Start time"=timestamp(0 s since 1904-01-01), "Trigger time"=timestamp(0 s since 1904-01-01), "End time"=timestamp(0 s since 1904-01-01)}, "Message type"=enum."New trigger"} ("Trigger message"), "Trigger timestamps"=w1128, "Message type"=w1127) -> (w1126:T15)
          }
          frame "In range" {
            # "We are still within recording trigger time period"
            n466 = Not(x=w1145) -> (.not. x?=w1144:bool)
            n467 = Compound Arithmetic op=AND(w1151, w1146, w1144) -> (w1147:bool)
            n468 = case shown="True" w1147 {
              tunnel: [w1154 w1161] -> w1149
              tunnel: w1152 -> [w1154 w1160]
              tunnel: [FALSE ("Mean above high threshold?") TRUE ("Mean above high threshold?")] -> w1150
              tunnel: w1148 -> [_ w1155]
              frame False {
                # "Audio mean has not been under threshold long enough.\nDo not update trigger time periods"
              }
              frame True {
                # "Audio mean amplitude was under threshold long enough (& not above high thresh)\nUpdate trigger stop time to be now!"
                n469 = Unbundle By Name(w1160) -> ("Trigger timestamps.Start time"=w1159:timestamp, "Trigger timestamps.Trigger time"=w1158:timestamp)
                n470 = Bundle By Name(cluster=w1160, "Trigger timestamps.Start time"=w1159, "Trigger timestamps.Trigger time"=w1158, "Trigger timestamps.End time"=w1155, "Message type"=Trigger_message."Updated trigger") -> (w1161:T15)
              }
            }
          }
        }
      }
    }
    n471 = Wait (ms)(milliseconds to wait=w992) -> ()  [unwired: 1 out]
    n472 = case shown="True" w993 {
      tunnel: w1006 -> [_ w1019]
      tunnel: w1001 -> [w1008 w1022]
      tunnel: [w1008 w1021] -> w1000
      tunnel: w999 -> [_ w1020]
      tunnel: w986 -> [w1007 w1014]
      tunnel: [w1007 w1014] -> w987
      frame False {
        # "No trigger detected"
      }
      frame True {
        # "New or updated trigger detected - signal write loops"
        n473 = Build Array(w1019, w1020) -> (w1016:refnum<queue>[])
        n474 = Unbundle By Name(w1014) -> ("Message type"=w1013:T14)
        n475 = Or(x="Enable audio write", y="Enable video write") -> (x .or. y?=w1015:bool)
        n476 = Build Array(w1015, w1015) -> (w1023:bool[])
        n477 = control-ref of="Events and errors"() -> (w1009:refnum<vi>)
        n478 = case shown="\"New trigger\", Default" w1013 {
          tunnel: ["New" ("New log entry") "updated" ("New log entry")] -> w1010
          frame "New trigger", Default {
            n479 = local read "New triggers sent"() -> (w1025:u32)
            n480 = Increment(x=w1025) -> (x+1=→"New triggers sent":u32)
          }
          frame "Updated trigger" {
            n481 = local read "Trigger updates sent"() -> (w1029:u32)
            n482 = Increment(x=w1029) -> (x+1=→"Trigger updates sent":u32)
          }
        }
        n483 = call "sendTriggersToWriteLoops.vi"("error in"=w1022, "Trigger message"=w1014, "Trigger queue enable array"=w1023, "Trigger queue array"=w1016) -> ("error out"=w1021:errorcluster)  [unwired: 7 in]
        n484 = Concatenate Strings("Write trigger signal sent - " ("New log entry"), w1010) -> (w1011:string)
        n485 = call "logEvent.vi"("New log entry"=w1011, "Text reference"=w1009) -> ()  [unwired: 9 in, 1 out]
      }
    }
    n486 = local read "STOP"() -> (w988:bool)
  }
  n487 = flat-sequence {
    tunnel: w20 -> [w1177]
    tunnel: w19 -> [w1176]
    tunnel: w18 -> [w1175]
    tunnel: w17 -> [w1174]
    tunnel: w16 -> [w1173]
    tunnel: w15 -> [w1172]
    tunnel: w14 -> [w1171]
    tunnel: w13 -> [w1169]
    tunnel: w12 -> [w1168]
    tunnel: w11 -> [w1167]
    tunnel: w10 -> [w1166]
    tunnel: w9 -> [w1165]
    tunnel: w8 -> [w1164]
    frame #0 {
      # "Clean up"
      n488 = call "IMAQ Dispose"("All Images? (No)"=TRUE) -> ("error out"=w1163:errorcluster)  [unwired: 5 in]
      n489 = Merge Errors(w1169, w1168, w1167, w1166, w1165, w1164, w1163) -> (w1162:errorcluster)
      n490 = call <vilib>:"Simple Error Handler.vi"("error in (no error)"=w1162) -> ()  [unwired: 4 in, 5 out]
      "Camera capture loop done" <- w1177
      "Audio capture loop done" <- w1176
      "Trigger detection loop done" <- w1175
      "Trigger out loop done" <- w1174
      "UI event loop done" <- w1173
      "Video write loop done" <- w1172
      "Mux loop done" <- w1171
    }
  }
